vi "Experiment header-bundle parameters section wise.vi"(6 "Logging queue element":T1={"Imaging Protocol"=enum."Live Imaging", "Number of Trials"=0, "Frame Size"=100, "# Averaged frames"=0, "Dwell time (us)"=0.1, "Index of Z-plane"=0, "Timelapse?"=FALSE, "Logging process is active"=FALSE, "Speed logging enabled"=FALSE, "tdms file ref"=refnum, "path"=path "", "Trial Number"=0, "Expected # points acquired"=FALSE, "Manually stopped"=FALSE, "Last trial"=FALSE, "Ch0 data"=[], "Ch1 data"=[], "Image Time"=[], "Continuous Time"=[], "Points acquired"={"Ch0 last trial"=0, "Ch1 last trial"=0, "All trials"=0}, "HW Timings File"=refnum} {"Frame Size" items=["100X100"=100, "128X128"=128, "200X200"=200, "256X256"=256, "512X512"=512, "1024x1024"=1024, "2048x2048"=2048]; "Dwell time (us)" format="%#.6g"}, 7 "Update header\ninterface cluster ?":bool, 8 "error in (no error)":errorcluster, 9 "Experiment data folder path":path, 10 "AOL_Globals":T22={"Imaging Protocol"=enum."AOL Z-Stack", "Number of POI"=0, "Number of Miniscans"=0, "Number of Trials"=0, "Number of Cycles "=0, "# Averaged Frames"=0, "Laser power (%)"=0, "Pockels (V)"=0.0, "Acquisition Length (sec)"=0.0, "Fill time (us)"=0.0, "POI Dwell time (us)"=0.0, "Miniscan Dwell time per pixel (us)"=0.0, "PMT 1"=0.0, "PMT 2"=0.0, "Back Apperture (mA)"=200.0, "Frame Size"=0, "Center Frequency"=0.0, "Field of View (norm)"=0.0, "DwellTime (us)"=0.0, "Wavelength (nm)"=0.0, "Zoom"=0.0, "AOL Z"=0.0, "AOL Mode"=enum."Raster", "GridXY"=0.0, "GridZ"=0.0, "TriggerPeriod (sec)"=0.0, "Number of Pixels in Miniscan"=0, "Experiment folder path"=path "", "X centre"=0.0, "Y centre"=0.0, "Angle (degrees)"=0.0, "Plane Mode"=0, "Threshold"=[], "Regenerate Chirps"=FALSE, "Rectangle ROI length (pixels)"=0, "Rectangle ROI height (pixels)"=0, "AOD fill"=4900, "StartupDelay"=0, "Samples Wait after Trigger"=5080, "Slip Cycle"=600000, "Add Cycle"=TRUE, "Functional Mode"=enum."Point", "Z Start"=0.0, "Z Stop"=0.0, "# Planes"=0} {"Plane Mode" items=["XY Plane", "XZ Plane", "YZ Plane", "arbitraryplane"]; "Frame Size" items=["100X100"=100, "128X128"=128, "200X200"=200, "256X256"=256, "512X512"=512, "1024x1024"=1024, "2048x2048"=2048]; "Back Apperture (mA)" format="%#.6g"; "Pockels (V)" format="%#.6g"; "PMT 2" format="%#.6g"; "PMT 1" format="%#.6g"; "Angle (degrees)" format="%#.6g"; "POI Dwell time (us)" format="%#.6g"}, 11 "Header file sections":T5=enum."GLOBAL PARAMETERS") -> (0 "error out":errorcluster, 3 "All header parameters in":T6 {"VOLUME IMAGING"."Plane Mode" items=["XY Plane", "XZ Plane", "YZ Plane", "arbitraryplane"]; "VOLUME IMAGING"."Basic Image meta data"."Frame Size" items=["100X100"=100, "128X128"=128, "200X200"=200, "256X256"=256, "512X512"=512, "1024x1024"=1024, "2048x2048"=2048]; "AOL Z-STACK"."Hdr Basic Image meta data"."Frame Size" items=["100X100"=100, "128X128"=128, "200X200"=200, "256X256"=256, "512X512"=512, "1024x1024"=1024, "2048x2048"=2048]; "MOTOR Z-STACK"."Hdr Basic Image meta data"."Frame Size" items=["100X100"=100, "128X128"=128, "200X200"=200, "256X256"=256, "512X512"=512, "1024x1024"=1024, "2048x2048"=2048]; "FUNCTIONAL IMAGING"."Plane Mode" items=["XY Plane", "XZ Plane", "YZ Plane", "arbitraryplane"]; "FUNCTIONAL IMAGING"."Basic Image meta data"."Frame Size" items=["100X100"=100, "128X128"=128, "200X200"=200, "256X256"=256, "512X512"=512, "1024x1024"=1024, "2048x2048"=2048]; "TIME SERIES"."Basic Image meta data"."Frame Size" items=["100X100"=100, "128X128"=128, "200X200"=200, "256X256"=256, "512X512"=512, "1024x1024"=1024, "2048x2048"=2048]})   [LabVIEW 2017]
uses:
  Typedefs/Controls/AOL_Globals.ctl
  Typedefs/Imaging Protocols enum.ctl
  Typedefs/Frame Size.ctl
  Typedefs/AOL modes.ctl
  Typedefs/Plane Mode.ctl
  Typedefs/Functional Mode.ctl
  Typedefs/Header parameters cluster-ALL.ctl
  Typedefs/Header subclusters/Header params -Login.ctl
  Typedefs/Header subclusters/Header params-Global Parameters.ctl
  Misc/Experiment Type.ctl
  Typedefs/Header subclusters/Header params-Imaging Modes.ctl
  Typedefs/Header subclusters/Header params-Time Series.ctl
  Typedefs/Header subclusters/Header params-Basic image meta data.ctl
  Typedefs/Header subclusters/Header params-Motor Z-stack.ctl
  Typedefs/Header subclusters/Header params-AOL Z-stack.ctl
  Typedefs/Header subclusters/Header params-Functional Imaging.ctl
  Typedefs/Header subclusters/Header params-Calibration Setup.ctl
  Typedefs/Header subclusters/Header params-statistics.ctl
  Misc/Biology Information.ctl
  Typedefs/Header file sections.ctl
  Typedefs/Logging queue element.ctl
  Typedefs/Acquired points count.ctl
  Typedefs/Header subclusters/Header params-Volume Imaging.ctl
  Typedefs/Header file interface module functions enum.ctl
  Global Variables/General Globals.vi
  User profiles code/Globals/gl_UsrProfiles globals.vi
  Global Variables/gl_UI Ctrl Refs.vi
  Peripherals Control/Pockels/Globals/gl_Pockels control globals.vi
  Configuration code/Calibration/Globals/gl_Calibration globals.vi
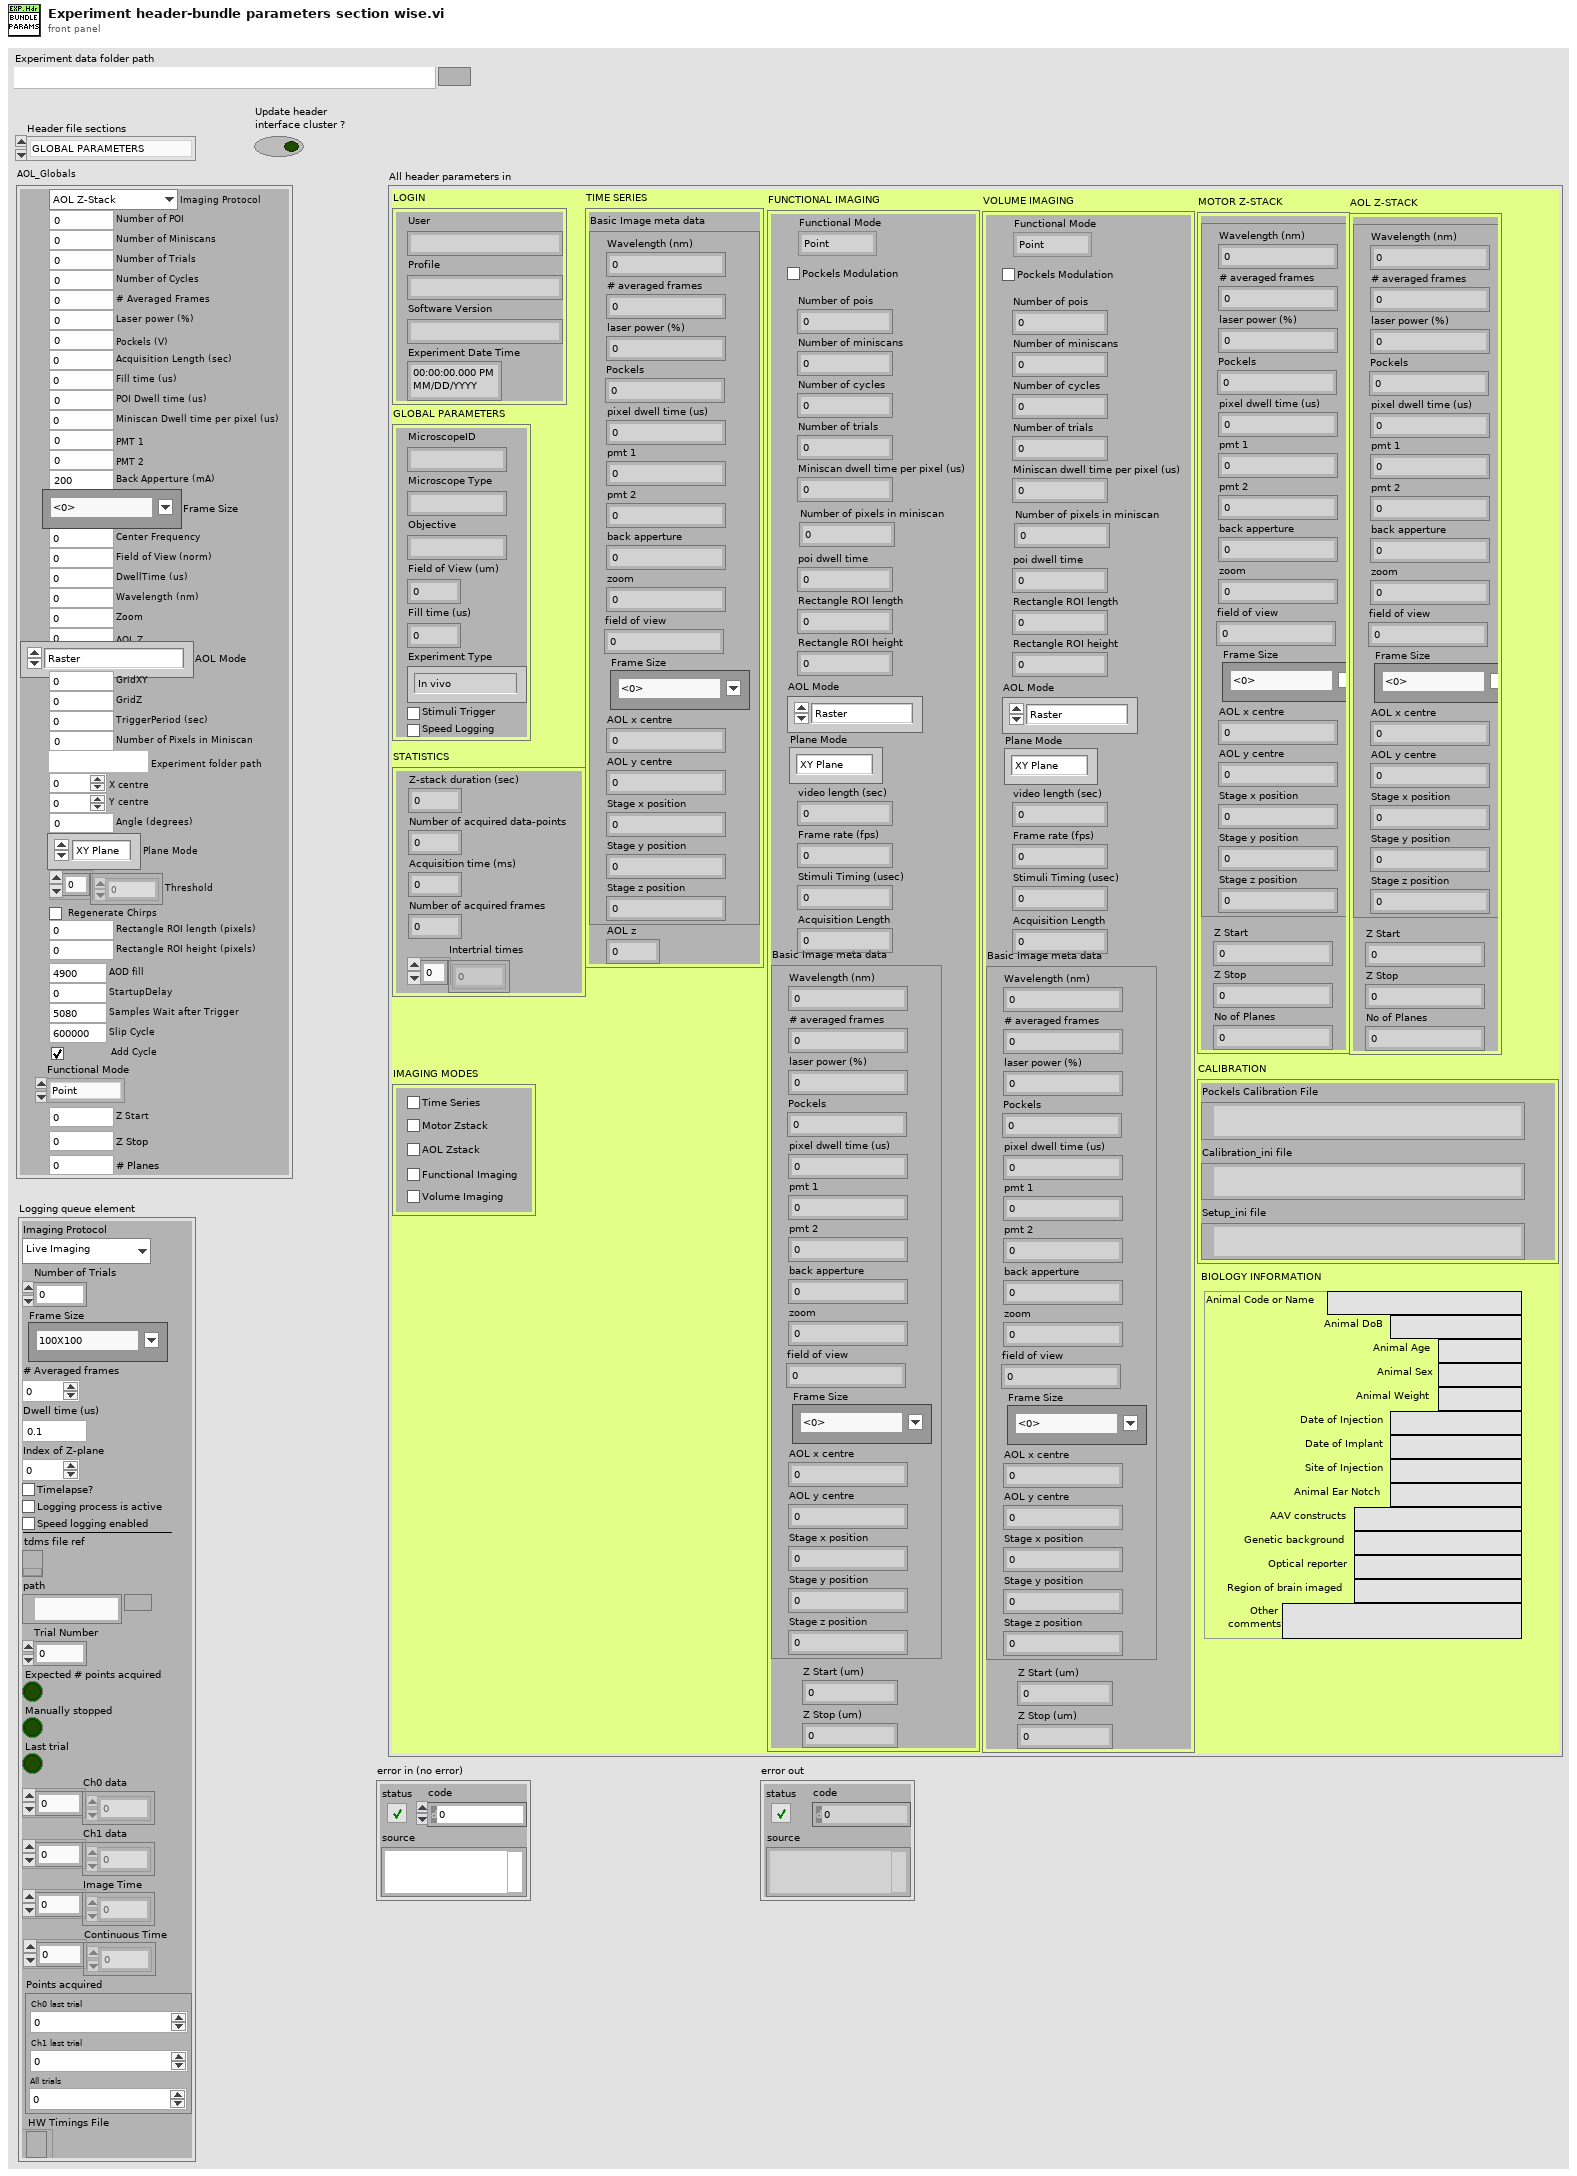
[diagram p1: front panel]
types:
  T1 = typedef "Logging queue element.ctl" = cluster{"Imaging Protocol":T2, "Number of Trials":u16, "Frame Size":T3, "# Averaged frames":u16, "Dwell time (us)":dbl, "Index of Z-plane":i32, "Timelapse?":bool, "Logging process is active":bool, "Speed logging enabled":bool, "tdms file ref":refnum<k34>, "path":path, "Trial Number":i32, "Expected # points acquired":bool, "Manually stopped":bool, "Last trial":bool, "Ch0 data":u32[], "Ch1 data":u32[], "Image Time":u64[], "Continuous Time":u64[], "Points acquired":T4, "HW Timings File":refnum<file>}
  T2 = typedef "Imaging Protocols enum.ctl" = enum16{"AOL Z-Stack", "Motor Z Stack", "Functional Acquisition", "Single Plane Acquisition", "Volume Acquisition", "Live Imaging", "Live Plane Imaging", "Live Volume Imaging"}
  T3 = typedef "Frame Size.ctl" = u16
  T4 = typedef "Acquired points count.ctl" = cluster{"Ch0 last trial":u64, "Ch1 last trial":u64, "All trials":u64}
  T5 = typedef "Header file sections.ctl" = enum16{"ALL SECTIONS", "LOGIN", "GLOBAL PARAMETERS", "IMAGING MODES", "TIME SERIES", "MOTOR Z-STACK", "AOL Z-STACK", "FUNCTIONAL IMAGING", "VOLUME IMAGING", "CALIBRATION", "STATISTICS", "BIOLOGY INFORMATION"}
  T6 = typedef "Header parameters cluster-ALL.ctl" = cluster{"LOGIN":T7, "GLOBAL PARAMETERS":T8, "IMAGING MODES":T10, "TIME SERIES":T11, "MOTOR Z-STACK ":T13, "AOL Z-STACK":T14, "FUNCTIONAL IMAGING":T15, "VOLUME IMAGING":T15, "CALIBRATION":T19, "STATISTICS":T20, "BIOLOGY INFORMATION":T21}
  T7 = typedef "Header params -Login.ctl" = cluster{"User":string, "Profile":string, "Software Version":string, "Experiment Date Time":timestamp}
  T8 = typedef "Header params-Global Parameters.ctl" = cluster{"MicroscopeID":string, "Microscope Type":string, "Objective":string, "Field of View (um)":dbl, "Fill time (us)":dbl, "Experiment Type":T9, "Stimuli Trigger":bool, "Speed Logging":bool}
  T9 = typedef "Experiment Type.ctl" = enum16{"In vivo", "In vitro", "Testing", "Calibration", "Other"}
  T10 = typedef "Header params-Imaging Modes.ctl" = cluster{"Time Series":bool, "Motor Zstack":bool, "AOL Zstack":bool, "Functional Imaging":bool, "Volume Imaging":bool}
  T11 = typedef "Header params-Time Series.ctl" = cluster{"Basic Image meta data":T12, "AOL z":dbl}
  T12 = typedef "Header params-Basic image meta data.ctl" = cluster{"Wavelength (nm)":dbl, "# averaged frames":dbl, "laser power (%)":dbl, "Pockels":dbl, "pixel dwell time (us)":dbl, "pmt 1":dbl, "pmt 2":dbl, "back apperture":dbl, "zoom":dbl, "field of view":dbl, "Frame Size":T3, "AOL x centre":dbl, "AOL y centre":dbl, "Stage x position":dbl, "Stage y position":dbl, "Stage z position":dbl}
  T13 = typedef "Header params-Motor Z-stack.ctl" = cluster{"Hdr Basic Image meta data":T12, "Z Start":dbl, "Z Stop":dbl, "No of Planes":i32}
  T14 = typedef "Header params-AOL Z-stack.ctl" = cluster{"Hdr Basic Image meta data":T12, "Z Start":dbl, "Z Stop":dbl, "No of Planes":i32}
  T15 = typedef "Header params-Functional Imaging.ctl" = cluster{"Functional Mode":T16, "Pockels Modulation":bool, "Number of pois":dbl, "Number of miniscans":dbl, "Number of cycles":dbl, "Number of trials":dbl, "Miniscan dwell time per pixel (us)":dbl, "Number of pixels in miniscan":dbl, "poi dwell time":dbl, "Rectangle ROI length":dbl, "Rectangle ROI height":dbl, "AOL Mode":T17, "Plane Mode":T18, "video length (sec)":dbl, "Frame rate (fps)":dbl, "Stimuli Timing (usec)":dbl, "Acquisition Length":dbl, "Basic Image meta data":T12, "Z Start (um)":dbl, "Z Stop (um)":dbl}
  T16 = typedef "Functional Mode.ctl" = enum16{"Point", "Line", "Patch", "Plane", "Volume"}
  T17 = typedef "AOL modes.ctl" = enum16{"Raster", "Structural", "Pointing", "Mini Scan", "Alignment"}
  T18 = typedef "Plane Mode.ctl" = u16
  T19 = typedef "Header params-Calibration Setup.ctl" = cluster{"Pockels Calibration File":path, "Calibration_ini file":path, "Setup_ini file":path}
  T20 = typedef "Header params-statistics.ctl" = cluster{"Z-stack duration (sec)":dbl, "Number of acquired data-points":dbl, "Acquisition time (ms)":dbl, "Number of acquired frames":dbl, "Intertrial times":dbl[]}
  T21 = typedef "Biology Information.ctl" = cluster{"Animal Code or Name":string, "Animal DoB":string, "Animal Age":string, "Animal Sex":string, "Animal Weight":string, "Date of Injection":string, "Date of Implant":string, "Site of Injection":string, "Animal Ear Notch":string, "AAV constructs":string, "Genetic background":string, "Optical reporter":string, "Region of brain imaged":string, "Other \ncomments":string}
  T22 = typedef "AOL_Globals.ctl" = cluster{"Imaging Protocol":T2, "Number of POI":u16, "Number of Miniscans":u16, "Number of Trials":u16, "Number of Cycles ":u64, "# Averaged Frames":u16, "Laser power (%)":u8, "Pockels (V)":dbl, "Acquisition Length (sec)":dbl, "Fill time (us)":dbl, "POI Dwell time (us)":dbl, "Miniscan Dwell time per pixel (us)":dbl, "PMT 1":dbl, "PMT 2":dbl, "Back Apperture (mA)":dbl, "Frame Size":T3, "Center Frequency":dbl, "Field of View (norm)":dbl, "DwellTime (us)":dbl, "Wavelength (nm)":dbl, "Zoom":dbl, "AOL Z":dbl, "AOL Mode":T17, "GridXY":dbl, "GridZ":dbl, "TriggerPeriod (sec)":dbl, "Number of Pixels in Miniscan":u16, "Experiment folder path":path, "X centre":dbl, "Y centre":dbl, "Angle (degrees)":dbl, "Plane Mode":T18, "Threshold":u16[], "Regenerate Chirps":bool, "Rectangle ROI length (pixels)":u16, "Rectangle ROI height (pixels)":u16, "AOD fill":u16, "StartupDelay":i32, "Samples Wait after Trigger":u16, "Slip Cycle":u32, "Add Cycle":bool, "Functional Mode":T16, "Z Start":dbl, "Z Stop":dbl, "# Planes":i32}
  T23 = typedef "Header params-Volume Imaging.ctl" = cluster{"Functional Mode":T16, "Pockels Modulation":bool, "Number of pois":dbl, "Number of miniscans":dbl, "Number of cycles":dbl, "Number of trials":dbl, "Miniscan dwell time per pixel (us)":dbl, "Number of pixels in miniscan":dbl, "poi dwell time":dbl, "Rectangle ROI length":dbl, "Rectangle ROI height":dbl, "AOL Mode":T17, "Plane Mode":T18, "video length (sec)":dbl, "Frame rate (fps)":dbl, "Stimuli Timing (usec)":dbl, "Acquisition Length":dbl, "Basic Image meta data":T12, "Z Start (um)":dbl, "Z Stop (um)":dbl}
  T24 = typedef "UI ctrl refs cluster.ctl" = cluster{"Top level VI path":path, "Top level VI ref":refnum<vi>, "User menu ref":refnum<k9>, "Sub Panel control":refnum<vi>, "Imaging Param Tab":refnum<vi>, "Occurrence-Start drivers":refnum<k4>, "Occurrence-Speed logging initialised":refnum<k4>, "Occurrence-XYZ stage initialised":refnum<k4>, "Exit button":refnum<vi>, "Status ind":refnum<vi>, "Set as origin":refnum<vi>, "Speed Logging":refnum<vi>, "Time Lapse":refnum<vi>, "Live Imaging":refnum<vi>, "AOL Z Stack":refnum<vi>, "Motor Z Stack":refnum<vi>, "Funct Acq button":refnum<vi>, "Hard Shutter":refnum<vi>, "Virtual Shutter":refnum<vi>, "Laser Power":refnum<vi>, "AOL Mode":refnum<vi>, "Frame Size":refnum<vi>, "Field of View":refnum<vi>, "Dwell Time":refnum<vi>, "Zoom":refnum<vi>, "AOL Z":refnum<vi>, "Objective":refnum<vi>, "Axis":refnum<vi>, "Paths & Names":refnum<vi>, "Experiment folder path (ind.)":refnum<vi>, "Last State (Ind.)":refnum<vi>, "Averages":refnum<vi>, "Angle (degrees)":refnum<vi>, "X centre":refnum<vi>, "Y centre":refnum<vi>, "Plane Mode":refnum<vi>, "# Planes":refnum<vi>, "Z Start":refnum<vi>, "Z Stop":refnum<vi>, "Z Step":refnum<vi>, "PMT 1":refnum<vi>, "PMT 2":refnum<vi>, "Stage XYZ Position":refnum<vi>, "Pockels@Z Start":refnum<vi>, "Pockels@Z Stop":refnum<vi>, "Obtain Z Start":refnum<vi>, "Obtain Z Stop":refnum<vi>, "Live stim.trig.period":refnum<vi>, "Live stim.trig.enable":refnum<vi>, "XY Stage Move":refnum<vi>, "Funct. Acq. Pockels Modulation":refnum<vi>, "Enable Video Recording":refnum<vi>, "Video Record-Live Imaging":refnum<vi>, "Video Record-Funct acq":refnum<vi>, "AOL Z-stack Chirps Ready (ind)":refnum<vi>, "Center freq ind (nm)":refnum<vi>, "Pickup mode (ind)":refnum<vi>, "Logging queue (ind)":refnum<vi>, "Back aperture power (ind.)":refnum<vi>, "Power after objective (ind.)":refnum<vi>, "Switch user":refnum<vi>, "Ls1 Conn. Status":refnum<vi>, "Ls1Tuning Status":refnum<vi>, "Ls1 Faults":refnum<vi>, "Ls1 Connection":refnum<vi>, "Ls1 Mode":refnum<vi>, "Ls1 POWER [mW]":refnum<vi>, "Ls1Shutter":refnum<vi>, "Ls1 Wavelength":refnum<vi>, "Ls1 Note":refnum<vi>, "Ls1 Confirm Wav":refnum<vi>, "Ls1 PreChrp Prism1":refnum<vi>, "Ls1 PreChrp Prism2":refnum<vi>, "Ls1 wav top Ind":refnum<vi>, "Ls1 power top Ind":refnum<vi>, "Ls1 Pump peak Hold":refnum<vi>, "Ls1 Status Ind":refnum<vi>, "Ls1 wav cancel":refnum<vi>, "Experiment Type":refnum<vi>, "Biology Information":refnum<vi>}
  T25 = typedef "Header file interface module functions enum.ctl" = enum16{"Load experiment header file", "Save experiment header file", "Clear stored values", "Read stored values", "Update specific value in memory", "Update values in memory"}
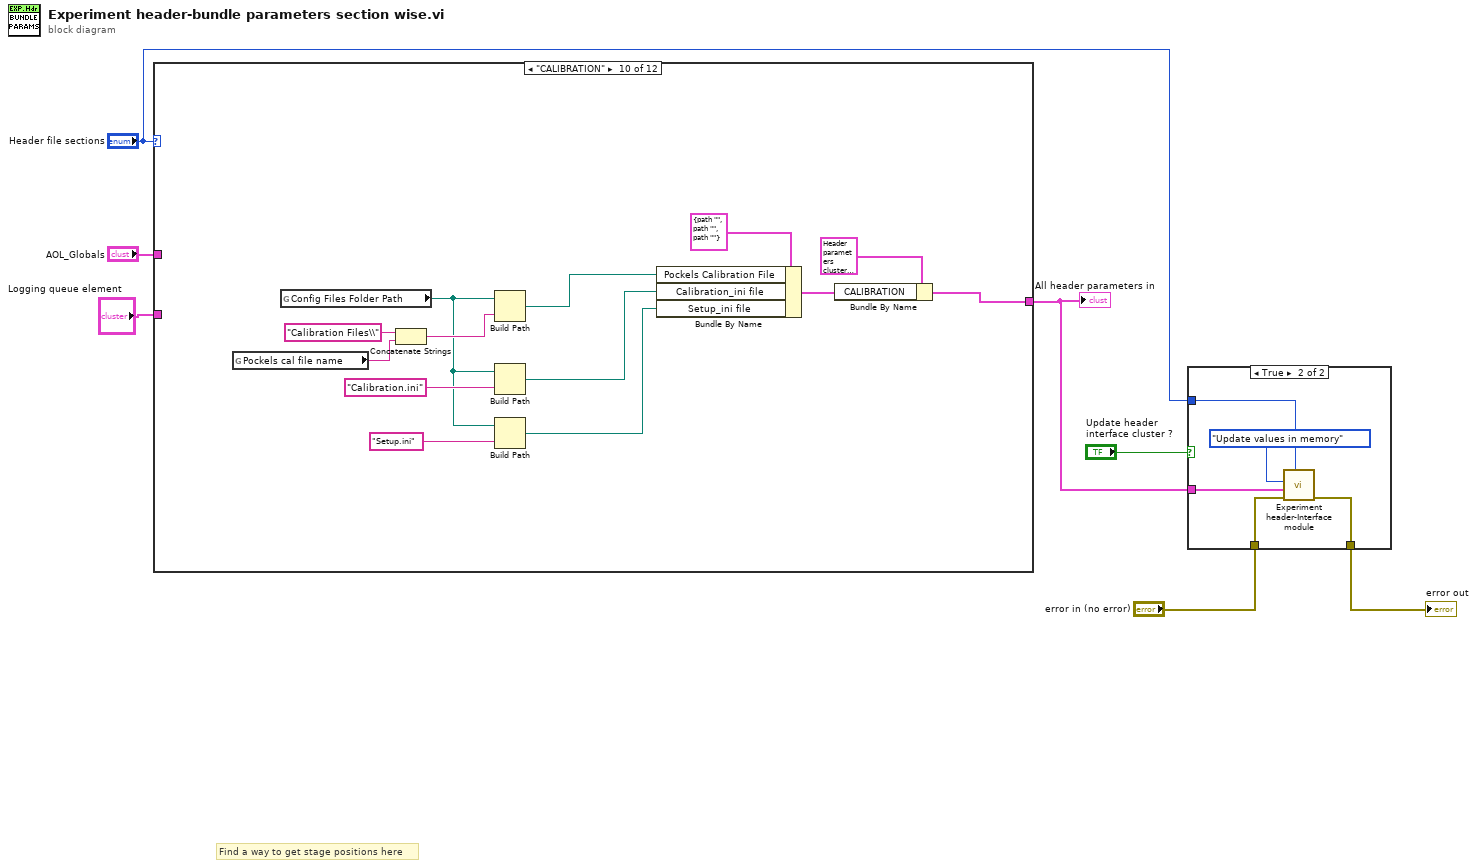
[diagram p0: block diagram]
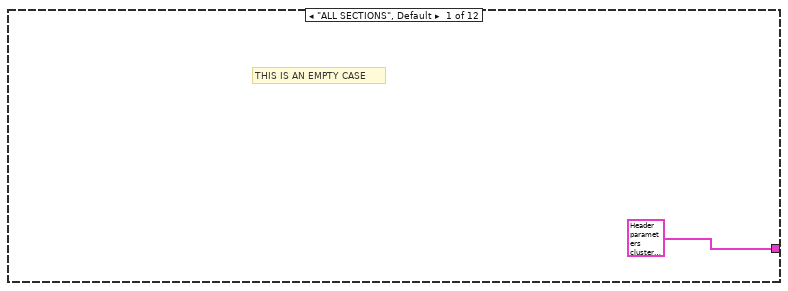
[diagram p3: hidden frame]
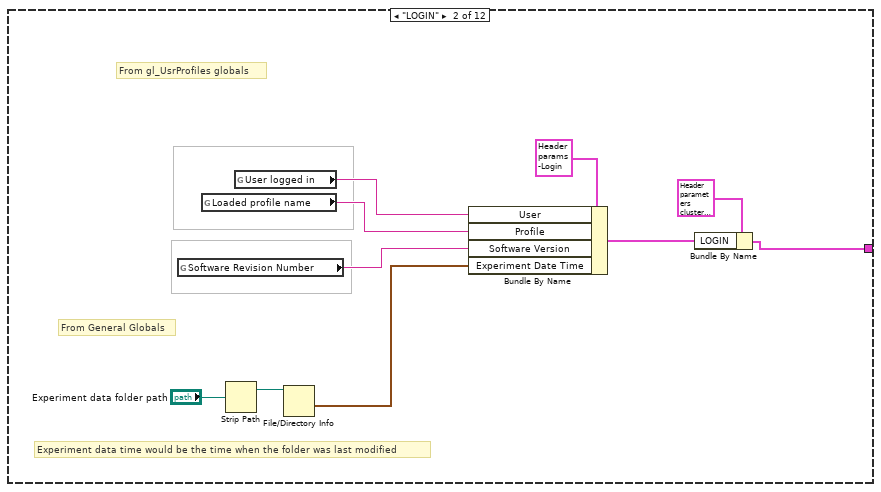
[diagram p4: hidden frame]
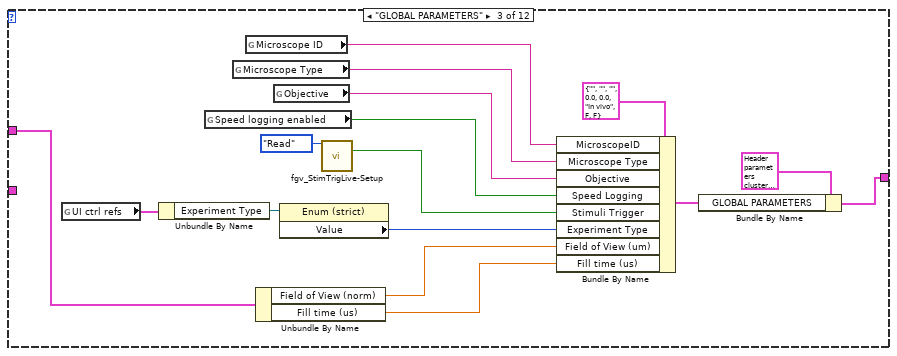
[diagram p5: hidden frame]
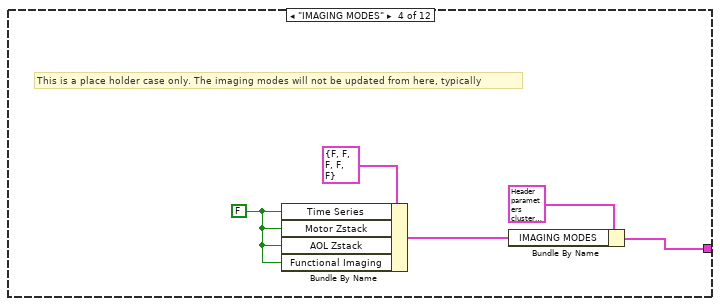
[diagram p6: hidden frame]
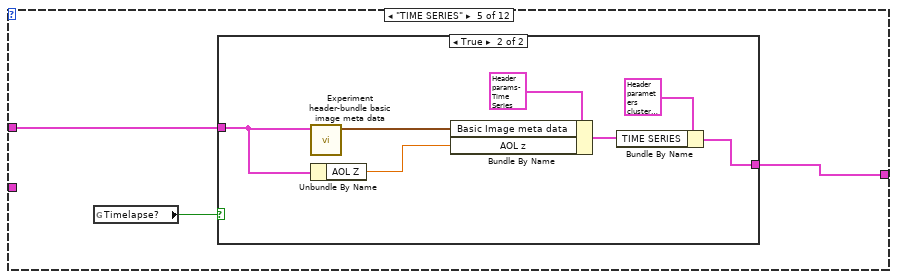
[diagram p7: hidden frame]
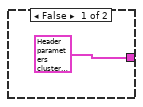
[diagram p8: hidden frame]
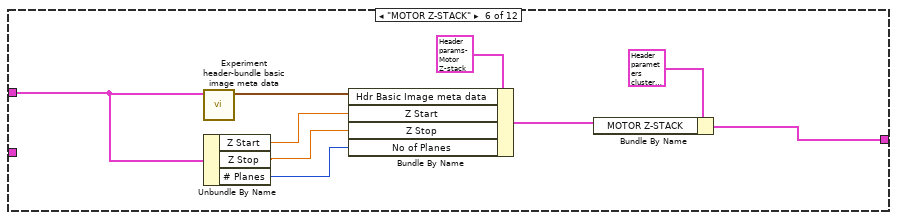
[diagram p9: hidden frame]
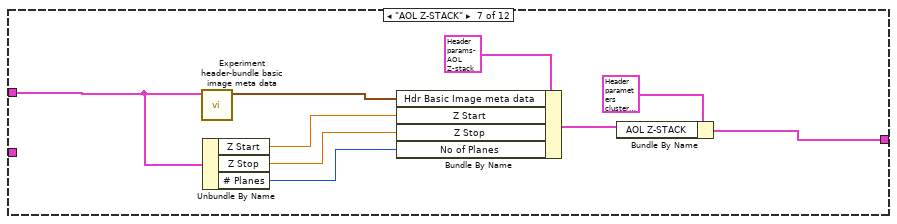
[diagram p10: hidden frame]
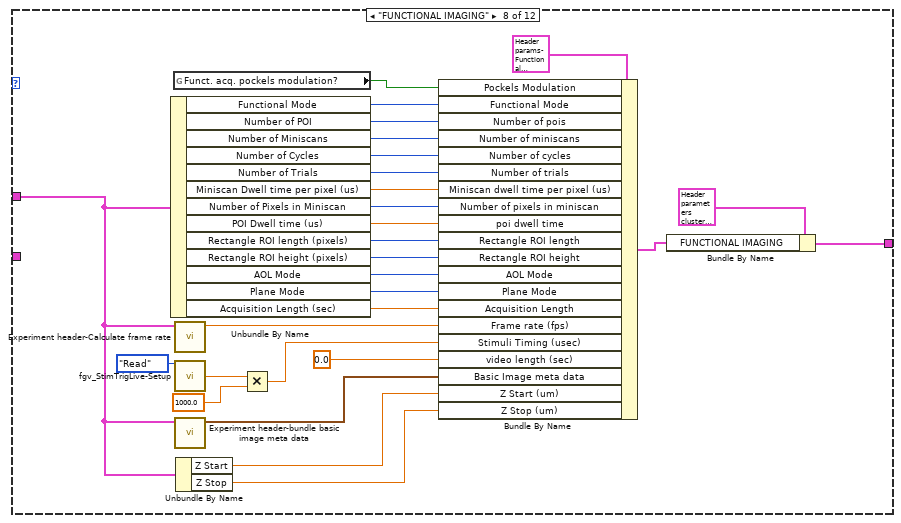
[diagram p11: hidden frame]
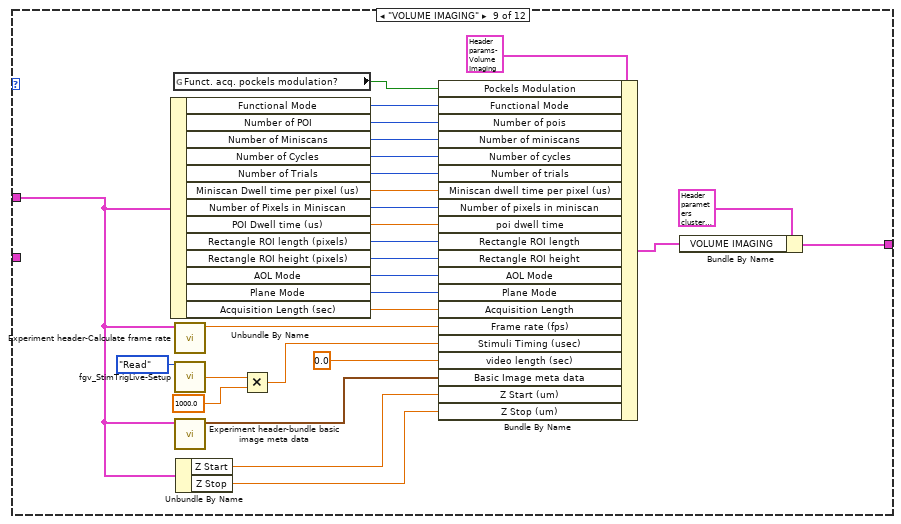
[diagram p12: hidden frame]
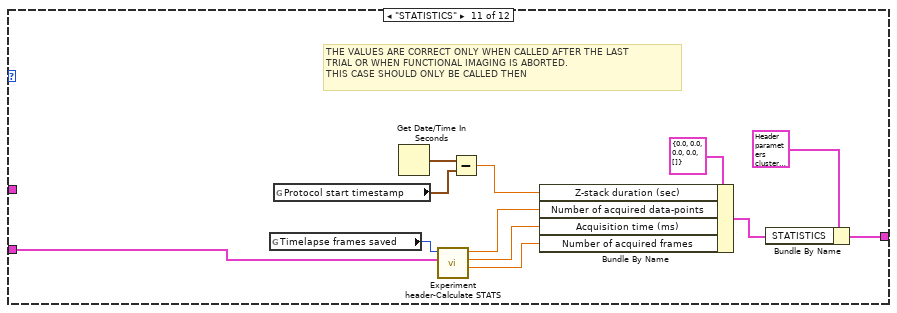
[diagram p13: hidden frame]
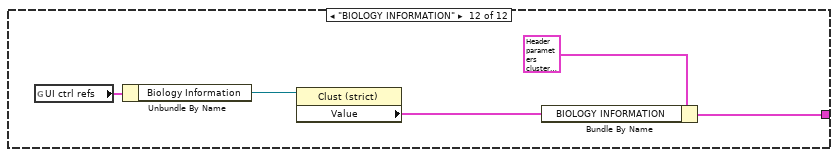
[diagram p14: hidden frame]
diagram:
  # "Find a way to get stage positions here"
  n1 = case shown="\"CALIBRATION\"" "Header file sections" {
    tunnel: "AOL_Globals" -> [_ _ w30 _ w41 w54 w63 w71 w100 _ _ _]
    tunnel: [T6 {"LOGIN"={"User"="Olympus  20X", "Profile"="", "Software Version"="", "Experiment Date Time"=timestamp(0 s since 1904-01-01)}, "GLOBAL PARAMETERS"={"MicroscopeID"="", "Microscope Type"="", "Objective"="", "Field of View (um)"=0.0, "Fill time (us)"=0.0, "Experiment Type"=enum."In vivo", "Stimuli Trigger"=FALSE, "Speed Logging"=FALSE}, "IMAGING MODES"={"Time Series"=FALSE, "Motor Zstack"=FALSE, "AOL Zstack"=FALSE, "Functional Imaging"=FALSE, "Volume Imaging"=FALSE}, "TIME SERIES"={"Basic Image meta data"={"Wavelength (nm)"=0.0, "# averaged frames"=0.0, "laser power (%)"=0.0, "Pockels"=0.0, "pixel dwell time (us)"=0.0, "pmt 1"=0.0, "pmt 2"=0.0, "back apperture"=0.0, "zoom"=0.0, "field of view"=0.0, "Frame Size"=0, "AOL x centre"=0.0, "AOL y centre"=0.0, "Stage x position"=0.0, "Stage y position"=0.0, "Stage z position"=0.0}, "AOL z"=0.0}, "MOTOR Z-STACK "={"Hdr Basic Image meta data"={"Wavelength (nm)"=0.0, "# averaged frames"=0.0, "laser power (%)"=0.0, "Pockels"=0.0, "pixel dwell time (us)"=0.0, "pmt 1"=0.0, "pmt 2"=0.0, "back apperture"=0.0, "zoom"=0.0, "field of view"=0.0, "Frame Size"=0, "AOL x centre"=0.0, "AOL y centre"=0.0, "Stage x position"=0.0, "Stage y position"=0.0, "Stage z position"=0.0}, "Z Start"=0.0, "Z Stop"=0.0, "No of Planes"=0}, "AOL Z-STACK"={"Hdr Basic Image meta data"={"Wavelength (nm)"=0.0, "# averaged frames"=0.0, "laser power (%)"=0.0, "Pockels"=0.0, "pixel dwell time (us)"=0.0, "pmt 1"=0.0, "pmt 2"=0.0, "back apperture"=0.0, "zoom"=0.0, "field of view"=0.0, "Frame Size"=0, "AOL x centre"=0.0, "AOL y centre"=0.0, "Stage x position"=0.0, "Stage y position"=0.0, "Stage z position"=0.0}, "Z Start"=0.0, "Z Stop"=0.0, "No of Planes"=0}, "FUNCTIONAL IMAGING"={"Functional Mode"=enum."Point", "Pockels Modulation"=FALSE, "Number of pois"=0.0, "Number of miniscans"=0.0, "Number of cycles"=0.0, "Number of trials"=0.0, "Miniscan dwell time per pixel (us)"=0.0, "Number of pixels in miniscan"=0.0, "poi dwell time"=0.0, "Rectangle ROI length"=0.0, "Rectangle ROI height"=0.0, "AOL Mode"=enum."Raster", "Plane Mode"=0, "video length (sec)"=0.0, "Frame rate (fps)"=0.0, "Stimuli Timing (usec)"=0.0, "Acquisition Length"=0.0, "Basic Image meta data"={"Wavelength (nm)"=0.0, "# averaged frames"=0.0, "laser power (%)"=0.0, "Pockels"=0.0, "pixel dwell time (us)"=0.0, "pmt 1"=0.0, "pmt 2"=0.0, "back apperture"=0.0, "zoom"=0.0, "field of view"=0.0, "Frame Size"=0, "AOL x centre"=0.0, "AOL y centre"=0.0, "Stage x position"=0.0, "Stage y position"=0.0, "Stage z position"=0.0}, "Z Start (um)"=0.0, "Z Stop (um)"=0.0}, "VOLUME IMAGING"={"Functional Mode"=enum."Point", "Pockels Modulation"=FALSE, "Number of pois"=0.0, "Number of miniscans"=0.0, "Number of cycles"=0.0, "Number of trials"=0.0, "Miniscan dwell time per pixel (us)"=0.0, "Number of pixels in miniscan"=0.0, "poi dwell time"=0.0, "Rectangle ROI length"=0.0, "Rectangle ROI height"=0.0, "AOL Mode"=enum."Raster", "Plane Mode"=0, "video length (sec)"=0.0, "Frame rate (fps)"=0.0, "Stimuli Timing (usec)"=0.0, "Acquisition Length"=0.0, "Basic Image meta data"={"Wavelength (nm)"=0.0, "# averaged frames"=0.0, "laser power (%)"=0.0, "Pockels"=0.0, "pixel dwell time (us)"=0.0, "pmt 1"=0.0, "pmt 2"=0.0, "back apperture"=0.0, "zoom"=0.0, "field of view"=0.0, "Frame Size"=0, "AOL x centre"=0.0, "AOL y centre"=0.0, "Stage x position"=0.0, "Stage y position"=0.0, "Stage z position"=0.0}, "Z Start (um)"=0.0, "Z Stop (um)"=0.0}, "CALIBRATION"={"Pockels Calibration File"=path "", "Calibration_ini file"=path "", "Setup_ini file"=path ""}, "STATISTICS"={"Z-stack duration (sec)"=0.0, "Number of acquired data-points"=0.0, "Acquisition time (ms)"=0.0, "Number of acquired frames"=0.0, "Intertrial times"=[]}, "BIOLOGY INFORMATION"={"Animal Code or Name"="", "Animal DoB"="", "Animal Age"="", "Animal Sex"="", "Animal Weight"="", "Date of Injection"="", "Date of Implant"="", "Site of Injection"="", "Animal Ear Notch"="", "AAV constructs"="", "Genetic background"="", "Optical reporter"="", "Region of brain imaged"="", "Other \ncomments"=""}} ("All header parameters in") w12 w19 w35 w42 w55 w66 w93 w122 w125 w148 w150] -> w6
    tunnel: "Logging queue element" -> [_ _ _ _ _ _ _ _ _ _ w146 _]
    frame "ALL SECTIONS", Default {
      # "THIS IS AN EMPTY CASE"
    }
    frame "LOGIN" {
      # "Experiment data time would be the time when the folder was last modified"
      # "From General Globals"
      # "From gl_UsrProfiles globals"
      n2 = global read "General Globals.vi" "Software Revision Number"() -> (w15:string)
      n3 = global read "gl_UsrProfiles globals.vi" "Loaded profile name"() -> (w16:string)
      n4 = Strip Path(path="Experiment data folder path") -> (stripped path=w10:path)  [unwired: 1 out]
      n5 = global read "gl_UsrProfiles globals.vi" "User logged in"() -> (w17:string)
      n6 = File/Directory Info(path=w10) -> (last mod=w9:timestamp)  [unwired: 1 in, 6 out]
      n7 = Bundle By Name(cluster=T7 {"User"="", "Profile"="", "Software Version"="", "Experiment Date Time"=timestamp(0 s since 1904-01-01)} ("LOGIN"), "User"=w17, "Profile"=w16, "Software Version"=w15, "Experiment Date Time"=w9) -> (w13:T7)
      n8 = Bundle By Name(cluster=T6 {"LOGIN"={"User"="Olympus  20X", "Profile"="", "Software Version"="", "Experiment Date Time"=timestamp(0 s since 1904-01-01)}, "GLOBAL PARAMETERS"={"MicroscopeID"="", "Microscope Type"="", "Objective"="", "Field of View (um)"=0.0, "Fill time (us)"=0.0, "Experiment Type"=enum."In vivo", "Stimuli Trigger"=FALSE, "Speed Logging"=FALSE}, "IMAGING MODES"={"Time Series"=FALSE, "Motor Zstack"=FALSE, "AOL Zstack"=FALSE, "Functional Imaging"=FALSE, "Volume Imaging"=FALSE}, "TIME SERIES"={"Basic Image meta data"={"Wavelength (nm)"=0.0, "# averaged frames"=0.0, "laser power (%)"=0.0, "Pockels"=0.0, "pixel dwell time (us)"=0.0, "pmt 1"=0.0, "pmt 2"=0.0, "back apperture"=0.0, "zoom"=0.0, "field of view"=0.0, "Frame Size"=0, "AOL x centre"=0.0, "AOL y centre"=0.0, "Stage x position"=0.0, "Stage y position"=0.0, "Stage z position"=0.0}, "AOL z"=0.0}, "MOTOR Z-STACK "={"Hdr Basic Image meta data"={"Wavelength (nm)"=0.0, "# averaged frames"=0.0, "laser power (%)"=0.0, "Pockels"=0.0, "pixel dwell time (us)"=0.0, "pmt 1"=0.0, "pmt 2"=0.0, "back apperture"=0.0, "zoom"=0.0, "field of view"=0.0, "Frame Size"=0, "AOL x centre"=0.0, "AOL y centre"=0.0, "Stage x position"=0.0, "Stage y position"=0.0, "Stage z position"=0.0}, "Z Start"=0.0, "Z Stop"=0.0, "No of Planes"=0}, "AOL Z-STACK"={"Hdr Basic Image meta data"={"Wavelength (nm)"=0.0, "# averaged frames"=0.0, "laser power (%)"=0.0, "Pockels"=0.0, "pixel dwell time (us)"=0.0, "pmt 1"=0.0, "pmt 2"=0.0, "back apperture"=0.0, "zoom"=0.0, "field of view"=0.0, "Frame Size"=0, "AOL x centre"=0.0, "AOL y centre"=0.0, "Stage x position"=0.0, "Stage y position"=0.0, "Stage z position"=0.0}, "Z Start"=0.0, "Z Stop"=0.0, "No of Planes"=0}, "FUNCTIONAL IMAGING"={"Functional Mode"=enum."Point", "Pockels Modulation"=FALSE, "Number of pois"=0.0, "Number of miniscans"=0.0, "Number of cycles"=0.0, "Number of trials"=0.0, "Miniscan dwell time per pixel (us)"=0.0, "Number of pixels in miniscan"=0.0, "poi dwell time"=0.0, "Rectangle ROI length"=0.0, "Rectangle ROI height"=0.0, "AOL Mode"=enum."Raster", "Plane Mode"=0, "video length (sec)"=0.0, "Frame rate (fps)"=0.0, "Stimuli Timing (usec)"=0.0, "Acquisition Length"=0.0, "Basic Image meta data"={"Wavelength (nm)"=0.0, "# averaged frames"=0.0, "laser power (%)"=0.0, "Pockels"=0.0, "pixel dwell time (us)"=0.0, "pmt 1"=0.0, "pmt 2"=0.0, "back apperture"=0.0, "zoom"=0.0, "field of view"=0.0, "Frame Size"=0, "AOL x centre"=0.0, "AOL y centre"=0.0, "Stage x position"=0.0, "Stage y position"=0.0, "Stage z position"=0.0}, "Z Start (um)"=0.0, "Z Stop (um)"=0.0}, "VOLUME IMAGING"={"Functional Mode"=enum."Point", "Pockels Modulation"=FALSE, "Number of pois"=0.0, "Number of miniscans"=0.0, "Number of cycles"=0.0, "Number of trials"=0.0, "Miniscan dwell time per pixel (us)"=0.0, "Number of pixels in miniscan"=0.0, "poi dwell time"=0.0, "Rectangle ROI length"=0.0, "Rectangle ROI height"=0.0, "AOL Mode"=enum."Raster", "Plane Mode"=0, "video length (sec)"=0.0, "Frame rate (fps)"=0.0, "Stimuli Timing (usec)"=0.0, "Acquisition Length"=0.0, "Basic Image meta data"={"Wavelength (nm)"=0.0, "# averaged frames"=0.0, "laser power (%)"=0.0, "Pockels"=0.0, "pixel dwell time (us)"=0.0, "pmt 1"=0.0, "pmt 2"=0.0, "back apperture"=0.0, "zoom"=0.0, "field of view"=0.0, "Frame Size"=0, "AOL x centre"=0.0, "AOL y centre"=0.0, "Stage x position"=0.0, "Stage y position"=0.0, "Stage z position"=0.0}, "Z Start (um)"=0.0, "Z Stop (um)"=0.0}, "CALIBRATION"={"Pockels Calibration File"=path "", "Calibration_ini file"=path "", "Setup_ini file"=path ""}, "STATISTICS"={"Z-stack duration (sec)"=0.0, "Number of acquired data-points"=0.0, "Acquisition time (ms)"=0.0, "Number of acquired frames"=0.0, "Intertrial times"=[]}, "BIOLOGY INFORMATION"={"Animal Code or Name"="", "Animal DoB"="", "Animal Age"="", "Animal Sex"="", "Animal Weight"="", "Date of Injection"="", "Date of Implant"="", "Site of Injection"="", "Animal Ear Notch"="", "AAV constructs"="", "Genetic background"="", "Optical reporter"="", "Region of brain imaged"="", "Other \ncomments"=""}} ("All header parameters in"), "LOGIN"=w13) -> (w12:T6)
    }
    frame "GLOBAL PARAMETERS" {
      n9 = global read "gl_UI Ctrl Refs.vi" "UI ctrl refs"() -> (w26:T24)
      n10 = Unbundle By Name(w26) -> ("Experiment Type"=w25:refnum<vi>)
      n11 = global read "General Globals.vi" "Speed logging enabled"() -> (w29:bool)
      n12 = global read "General Globals.vi" "Microscope Type"() -> (w32:string)
      n13 = global read "General Globals.vi" "Microscope ID"() -> (w33:string)
      n14 = Unbundle By Name(w30) -> ("Field of View (norm)"=w23:dbl, "Fill time (us)"=w22:dbl)
      n15 = global read "General Globals.vi" "Objective"() -> (w31:string)
      n16 = property class="Enum (strict)"(reference=w25) -> ("Value"=w24:T9)  [unwired: 1 in, 2 out]
      n17 = call "fgv_StimTrigLive-Setup.vi"("Function"=enum16{"Intialize", "Write", "Read", "Clear"}."Read") -> ("Live stim.trig.enable"=w27:bool)  [unwired: 11 in, 3 out]
      n18 = Bundle By Name(cluster=T8 {"MicroscopeID"="", "Microscope Type"="", "Objective"="", "Field of View (um)"=0.0, "Fill time (us)"=0.0, "Experiment Type"=enum."In vivo", "Stimuli Trigger"=FALSE, "Speed Logging"=FALSE} ("GLOBAL PARAMETERS"), "MicroscopeID"=w33, "Microscope Type"=w32, "Objective"=w31, "Speed Logging"=w29, "Stimuli Trigger"=w27, "Experiment Type"=w24, "Field of View (um)"=w23, "Fill time (us)"=w22) -> (w20:T8)
      n19 = Bundle By Name(cluster=T6 {"LOGIN"={"User"="Olympus  20X", "Profile"="", "Software Version"="", "Experiment Date Time"=timestamp(0 s since 1904-01-01)}, "GLOBAL PARAMETERS"={"MicroscopeID"="", "Microscope Type"="", "Objective"="", "Field of View (um)"=0.0, "Fill time (us)"=0.0, "Experiment Type"=enum."In vivo", "Stimuli Trigger"=FALSE, "Speed Logging"=FALSE}, "IMAGING MODES"={"Time Series"=FALSE, "Motor Zstack"=FALSE, "AOL Zstack"=FALSE, "Functional Imaging"=FALSE, "Volume Imaging"=FALSE}, "TIME SERIES"={"Basic Image meta data"={"Wavelength (nm)"=0.0, "# averaged frames"=0.0, "laser power (%)"=0.0, "Pockels"=0.0, "pixel dwell time (us)"=0.0, "pmt 1"=0.0, "pmt 2"=0.0, "back apperture"=0.0, "zoom"=0.0, "field of view"=0.0, "Frame Size"=0, "AOL x centre"=0.0, "AOL y centre"=0.0, "Stage x position"=0.0, "Stage y position"=0.0, "Stage z position"=0.0}, "AOL z"=0.0}, "MOTOR Z-STACK "={"Hdr Basic Image meta data"={"Wavelength (nm)"=0.0, "# averaged frames"=0.0, "laser power (%)"=0.0, "Pockels"=0.0, "pixel dwell time (us)"=0.0, "pmt 1"=0.0, "pmt 2"=0.0, "back apperture"=0.0, "zoom"=0.0, "field of view"=0.0, "Frame Size"=0, "AOL x centre"=0.0, "AOL y centre"=0.0, "Stage x position"=0.0, "Stage y position"=0.0, "Stage z position"=0.0}, "Z Start"=0.0, "Z Stop"=0.0, "No of Planes"=0}, "AOL Z-STACK"={"Hdr Basic Image meta data"={"Wavelength (nm)"=0.0, "# averaged frames"=0.0, "laser power (%)"=0.0, "Pockels"=0.0, "pixel dwell time (us)"=0.0, "pmt 1"=0.0, "pmt 2"=0.0, "back apperture"=0.0, "zoom"=0.0, "field of view"=0.0, "Frame Size"=0, "AOL x centre"=0.0, "AOL y centre"=0.0, "Stage x position"=0.0, "Stage y position"=0.0, "Stage z position"=0.0}, "Z Start"=0.0, "Z Stop"=0.0, "No of Planes"=0}, "FUNCTIONAL IMAGING"={"Functional Mode"=enum."Point", "Pockels Modulation"=FALSE, "Number of pois"=0.0, "Number of miniscans"=0.0, "Number of cycles"=0.0, "Number of trials"=0.0, "Miniscan dwell time per pixel (us)"=0.0, "Number of pixels in miniscan"=0.0, "poi dwell time"=0.0, "Rectangle ROI length"=0.0, "Rectangle ROI height"=0.0, "AOL Mode"=enum."Raster", "Plane Mode"=0, "video length (sec)"=0.0, "Frame rate (fps)"=0.0, "Stimuli Timing (usec)"=0.0, "Acquisition Length"=0.0, "Basic Image meta data"={"Wavelength (nm)"=0.0, "# averaged frames"=0.0, "laser power (%)"=0.0, "Pockels"=0.0, "pixel dwell time (us)"=0.0, "pmt 1"=0.0, "pmt 2"=0.0, "back apperture"=0.0, "zoom"=0.0, "field of view"=0.0, "Frame Size"=0, "AOL x centre"=0.0, "AOL y centre"=0.0, "Stage x position"=0.0, "Stage y position"=0.0, "Stage z position"=0.0}, "Z Start (um)"=0.0, "Z Stop (um)"=0.0}, "VOLUME IMAGING"={"Functional Mode"=enum."Point", "Pockels Modulation"=FALSE, "Number of pois"=0.0, "Number of miniscans"=0.0, "Number of cycles"=0.0, "Number of trials"=0.0, "Miniscan dwell time per pixel (us)"=0.0, "Number of pixels in miniscan"=0.0, "poi dwell time"=0.0, "Rectangle ROI length"=0.0, "Rectangle ROI height"=0.0, "AOL Mode"=enum."Raster", "Plane Mode"=0, "video length (sec)"=0.0, "Frame rate (fps)"=0.0, "Stimuli Timing (usec)"=0.0, "Acquisition Length"=0.0, "Basic Image meta data"={"Wavelength (nm)"=0.0, "# averaged frames"=0.0, "laser power (%)"=0.0, "Pockels"=0.0, "pixel dwell time (us)"=0.0, "pmt 1"=0.0, "pmt 2"=0.0, "back apperture"=0.0, "zoom"=0.0, "field of view"=0.0, "Frame Size"=0, "AOL x centre"=0.0, "AOL y centre"=0.0, "Stage x position"=0.0, "Stage y position"=0.0, "Stage z position"=0.0}, "Z Start (um)"=0.0, "Z Stop (um)"=0.0}, "CALIBRATION"={"Pockels Calibration File"=path "", "Calibration_ini file"=path "", "Setup_ini file"=path ""}, "STATISTICS"={"Z-stack duration (sec)"=0.0, "Number of acquired data-points"=0.0, "Acquisition time (ms)"=0.0, "Number of acquired frames"=0.0, "Intertrial times"=[]}, "BIOLOGY INFORMATION"={"Animal Code or Name"="", "Animal DoB"="", "Animal Age"="", "Animal Sex"="", "Animal Weight"="", "Date of Injection"="", "Date of Implant"="", "Site of Injection"="", "Animal Ear Notch"="", "AAV constructs"="", "Genetic background"="", "Optical reporter"="", "Region of brain imaged"="", "Other \ncomments"=""}} ("All header parameters in"), "GLOBAL PARAMETERS"=w20) -> (w19:T6)
    }
    frame "IMAGING MODES" {
      w38 = FALSE ("Time Series")
      # "This is a place holder case only. The imaging modes will not be updated from here, typically"
      n20 = Bundle By Name(cluster=T10 {"Time Series"=FALSE, "Motor Zstack"=FALSE, "AOL Zstack"=FALSE, "Functional Imaging"=FALSE, "Volume Imaging"=FALSE} ("IMAGING MODES"), "Time Series"=w38, "Motor Zstack"=w38, "AOL Zstack"=w38, "Functional Imaging"=w38) -> (w36:T10)
      n21 = Bundle By Name(cluster=T6 {"LOGIN"={"User"="Olympus  20X", "Profile"="", "Software Version"="", "Experiment Date Time"=timestamp(0 s since 1904-01-01)}, "GLOBAL PARAMETERS"={"MicroscopeID"="", "Microscope Type"="", "Objective"="", "Field of View (um)"=0.0, "Fill time (us)"=0.0, "Experiment Type"=enum."In vivo", "Stimuli Trigger"=FALSE, "Speed Logging"=FALSE}, "IMAGING MODES"={"Time Series"=FALSE, "Motor Zstack"=FALSE, "AOL Zstack"=FALSE, "Functional Imaging"=FALSE, "Volume Imaging"=FALSE}, "TIME SERIES"={"Basic Image meta data"={"Wavelength (nm)"=0.0, "# averaged frames"=0.0, "laser power (%)"=0.0, "Pockels"=0.0, "pixel dwell time (us)"=0.0, "pmt 1"=0.0, "pmt 2"=0.0, "back apperture"=0.0, "zoom"=0.0, "field of view"=0.0, "Frame Size"=0, "AOL x centre"=0.0, "AOL y centre"=0.0, "Stage x position"=0.0, "Stage y position"=0.0, "Stage z position"=0.0}, "AOL z"=0.0}, "MOTOR Z-STACK "={"Hdr Basic Image meta data"={"Wavelength (nm)"=0.0, "# averaged frames"=0.0, "laser power (%)"=0.0, "Pockels"=0.0, "pixel dwell time (us)"=0.0, "pmt 1"=0.0, "pmt 2"=0.0, "back apperture"=0.0, "zoom"=0.0, "field of view"=0.0, "Frame Size"=0, "AOL x centre"=0.0, "AOL y centre"=0.0, "Stage x position"=0.0, "Stage y position"=0.0, "Stage z position"=0.0}, "Z Start"=0.0, "Z Stop"=0.0, "No of Planes"=0}, "AOL Z-STACK"={"Hdr Basic Image meta data"={"Wavelength (nm)"=0.0, "# averaged frames"=0.0, "laser power (%)"=0.0, "Pockels"=0.0, "pixel dwell time (us)"=0.0, "pmt 1"=0.0, "pmt 2"=0.0, "back apperture"=0.0, "zoom"=0.0, "field of view"=0.0, "Frame Size"=0, "AOL x centre"=0.0, "AOL y centre"=0.0, "Stage x position"=0.0, "Stage y position"=0.0, "Stage z position"=0.0}, "Z Start"=0.0, "Z Stop"=0.0, "No of Planes"=0}, "FUNCTIONAL IMAGING"={"Functional Mode"=enum."Point", "Pockels Modulation"=FALSE, "Number of pois"=0.0, "Number of miniscans"=0.0, "Number of cycles"=0.0, "Number of trials"=0.0, "Miniscan dwell time per pixel (us)"=0.0, "Number of pixels in miniscan"=0.0, "poi dwell time"=0.0, "Rectangle ROI length"=0.0, "Rectangle ROI height"=0.0, "AOL Mode"=enum."Raster", "Plane Mode"=0, "video length (sec)"=0.0, "Frame rate (fps)"=0.0, "Stimuli Timing (usec)"=0.0, "Acquisition Length"=0.0, "Basic Image meta data"={"Wavelength (nm)"=0.0, "# averaged frames"=0.0, "laser power (%)"=0.0, "Pockels"=0.0, "pixel dwell time (us)"=0.0, "pmt 1"=0.0, "pmt 2"=0.0, "back apperture"=0.0, "zoom"=0.0, "field of view"=0.0, "Frame Size"=0, "AOL x centre"=0.0, "AOL y centre"=0.0, "Stage x position"=0.0, "Stage y position"=0.0, "Stage z position"=0.0}, "Z Start (um)"=0.0, "Z Stop (um)"=0.0}, "VOLUME IMAGING"={"Functional Mode"=enum."Point", "Pockels Modulation"=FALSE, "Number of pois"=0.0, "Number of miniscans"=0.0, "Number of cycles"=0.0, "Number of trials"=0.0, "Miniscan dwell time per pixel (us)"=0.0, "Number of pixels in miniscan"=0.0, "poi dwell time"=0.0, "Rectangle ROI length"=0.0, "Rectangle ROI height"=0.0, "AOL Mode"=enum."Raster", "Plane Mode"=0, "video length (sec)"=0.0, "Frame rate (fps)"=0.0, "Stimuli Timing (usec)"=0.0, "Acquisition Length"=0.0, "Basic Image meta data"={"Wavelength (nm)"=0.0, "# averaged frames"=0.0, "laser power (%)"=0.0, "Pockels"=0.0, "pixel dwell time (us)"=0.0, "pmt 1"=0.0, "pmt 2"=0.0, "back apperture"=0.0, "zoom"=0.0, "field of view"=0.0, "Frame Size"=0, "AOL x centre"=0.0, "AOL y centre"=0.0, "Stage x position"=0.0, "Stage y position"=0.0, "Stage z position"=0.0}, "Z Start (um)"=0.0, "Z Stop (um)"=0.0}, "CALIBRATION"={"Pockels Calibration File"=path "", "Calibration_ini file"=path "", "Setup_ini file"=path ""}, "STATISTICS"={"Z-stack duration (sec)"=0.0, "Number of acquired data-points"=0.0, "Acquisition time (ms)"=0.0, "Number of acquired frames"=0.0, "Intertrial times"=[]}, "BIOLOGY INFORMATION"={"Animal Code or Name"="", "Animal DoB"="", "Animal Age"="", "Animal Sex"="", "Animal Weight"="", "Date of Injection"="", "Date of Implant"="", "Site of Injection"="", "Animal Ear Notch"="", "AAV constructs"="", "Genetic background"="", "Optical reporter"="", "Region of brain imaged"="", "Other \ncomments"=""}} ("All header parameters in"), "IMAGING MODES"=w36) -> (w35:T6)
    }
    frame "TIME SERIES" {
      n22 = global read "General Globals.vi" "Timelapse?"() -> (w40:bool)
      n23 = case shown="True" w40 {
        tunnel: [T6 {"LOGIN"={"User"="Olympus  20X", "Profile"="", "Software Version"="", "Experiment Date Time"=timestamp(0 s since 1904-01-01)}, "GLOBAL PARAMETERS"={"MicroscopeID"="", "Microscope Type"="", "Objective"="", "Field of View (um)"=0.0, "Fill time (us)"=0.0, "Experiment Type"=enum."In vivo", "Stimuli Trigger"=FALSE, "Speed Logging"=FALSE}, "IMAGING MODES"={"Time Series"=FALSE, "Motor Zstack"=FALSE, "AOL Zstack"=FALSE, "Functional Imaging"=FALSE, "Volume Imaging"=FALSE}, "TIME SERIES"={"Basic Image meta data"={"Wavelength (nm)"=0.0, "# averaged frames"=0.0, "laser power (%)"=0.0, "Pockels"=0.0, "pixel dwell time (us)"=0.0, "pmt 1"=0.0, "pmt 2"=0.0, "back apperture"=0.0, "zoom"=0.0, "field of view"=0.0, "Frame Size"=0, "AOL x centre"=0.0, "AOL y centre"=0.0, "Stage x position"=0.0, "Stage y position"=0.0, "Stage z position"=0.0}, "AOL z"=0.0}, "MOTOR Z-STACK "={"Hdr Basic Image meta data"={"Wavelength (nm)"=0.0, "# averaged frames"=0.0, "laser power (%)"=0.0, "Pockels"=0.0, "pixel dwell time (us)"=0.0, "pmt 1"=0.0, "pmt 2"=0.0, "back apperture"=0.0, "zoom"=0.0, "field of view"=0.0, "Frame Size"=0, "AOL x centre"=0.0, "AOL y centre"=0.0, "Stage x position"=0.0, "Stage y position"=0.0, "Stage z position"=0.0}, "Z Start"=0.0, "Z Stop"=0.0, "No of Planes"=0}, "AOL Z-STACK"={"Hdr Basic Image meta data"={"Wavelength (nm)"=0.0, "# averaged frames"=0.0, "laser power (%)"=0.0, "Pockels"=0.0, "pixel dwell time (us)"=0.0, "pmt 1"=0.0, "pmt 2"=0.0, "back apperture"=0.0, "zoom"=0.0, "field of view"=0.0, "Frame Size"=0, "AOL x centre"=0.0, "AOL y centre"=0.0, "Stage x position"=0.0, "Stage y position"=0.0, "Stage z position"=0.0}, "Z Start"=0.0, "Z Stop"=0.0, "No of Planes"=0}, "FUNCTIONAL IMAGING"={"Functional Mode"=enum."Point", "Pockels Modulation"=FALSE, "Number of pois"=0.0, "Number of miniscans"=0.0, "Number of cycles"=0.0, "Number of trials"=0.0, "Miniscan dwell time per pixel (us)"=0.0, "Number of pixels in miniscan"=0.0, "poi dwell time"=0.0, "Rectangle ROI length"=0.0, "Rectangle ROI height"=0.0, "AOL Mode"=enum."Raster", "Plane Mode"=0, "video length (sec)"=0.0, "Frame rate (fps)"=0.0, "Stimuli Timing (usec)"=0.0, "Acquisition Length"=0.0, "Basic Image meta data"={"Wavelength (nm)"=0.0, "# averaged frames"=0.0, "laser power (%)"=0.0, "Pockels"=0.0, "pixel dwell time (us)"=0.0, "pmt 1"=0.0, "pmt 2"=0.0, "back apperture"=0.0, "zoom"=0.0, "field of view"=0.0, "Frame Size"=0, "AOL x centre"=0.0, "AOL y centre"=0.0, "Stage x position"=0.0, "Stage y position"=0.0, "Stage z position"=0.0}, "Z Start (um)"=0.0, "Z Stop (um)"=0.0}, "VOLUME IMAGING"={"Functional Mode"=enum."Point", "Pockels Modulation"=FALSE, "Number of pois"=0.0, "Number of miniscans"=0.0, "Number of cycles"=0.0, "Number of trials"=0.0, "Miniscan dwell time per pixel (us)"=0.0, "Number of pixels in miniscan"=0.0, "poi dwell time"=0.0, "Rectangle ROI length"=0.0, "Rectangle ROI height"=0.0, "AOL Mode"=enum."Raster", "Plane Mode"=0, "video length (sec)"=0.0, "Frame rate (fps)"=0.0, "Stimuli Timing (usec)"=0.0, "Acquisition Length"=0.0, "Basic Image meta data"={"Wavelength (nm)"=0.0, "# averaged frames"=0.0, "laser power (%)"=0.0, "Pockels"=0.0, "pixel dwell time (us)"=0.0, "pmt 1"=0.0, "pmt 2"=0.0, "back apperture"=0.0, "zoom"=0.0, "field of view"=0.0, "Frame Size"=0, "AOL x centre"=0.0, "AOL y centre"=0.0, "Stage x position"=0.0, "Stage y position"=0.0, "Stage z position"=0.0}, "Z Start (um)"=0.0, "Z Stop (um)"=0.0}, "CALIBRATION"={"Pockels Calibration File"=path "", "Calibration_ini file"=path "", "Setup_ini file"=path ""}, "STATISTICS"={"Z-stack duration (sec)"=0.0, "Number of acquired data-points"=0.0, "Acquisition time (ms)"=0.0, "Number of acquired frames"=0.0, "Intertrial times"=[]}, "BIOLOGY INFORMATION"={"Animal Code or Name"="", "Animal DoB"="", "Animal Age"="", "Animal Sex"="", "Animal Weight"="", "Date of Injection"="", "Date of Implant"="", "Site of Injection"="", "Animal Ear Notch"="", "AAV constructs"="", "Genetic background"="", "Optical reporter"="", "Region of brain imaged"="", "Other \ncomments"=""}} ("All header parameters in") w46] -> w42
        tunnel: w41 -> [_ w45]
        frame False {
        }
        frame True {
          n24 = call "Experiment header-bundle basic image meta data.vi"("AOL_Globals"=w45) -> ("Basic image meta-data"=w50:T12)  [unwired: 10 in]
          n25 = Unbundle By Name(w45) -> ("AOL Z"=w44:dbl)
          n26 = Bundle By Name(cluster=T11 {"Basic Image meta data"={"Wavelength (nm)"=0.0, "# averaged frames"=0.0, "laser power (%)"=0.0, "Pockels"=0.0, "pixel dwell time (us)"=0.0, "pmt 1"=0.0, "pmt 2"=0.0, "back apperture"=0.0, "zoom"=0.0, "field of view"=0.0, "Frame Size"=0, "AOL x centre"=0.0, "AOL y centre"=0.0, "Stage x position"=0.0, "Stage y position"=0.0, "Stage z position"=0.0}, "AOL z"=0.0} ("TIME SERIES"), "Basic Image meta data"=w50, "AOL z"=w44) -> (w47:T11)
          n27 = Bundle By Name(cluster=T6 {"LOGIN"={"User"="Olympus  20X", "Profile"="", "Software Version"="", "Experiment Date Time"=timestamp(0 s since 1904-01-01)}, "GLOBAL PARAMETERS"={"MicroscopeID"="", "Microscope Type"="", "Objective"="", "Field of View (um)"=0.0, "Fill time (us)"=0.0, "Experiment Type"=enum."In vivo", "Stimuli Trigger"=FALSE, "Speed Logging"=FALSE}, "IMAGING MODES"={"Time Series"=FALSE, "Motor Zstack"=FALSE, "AOL Zstack"=FALSE, "Functional Imaging"=FALSE, "Volume Imaging"=FALSE}, "TIME SERIES"={"Basic Image meta data"={"Wavelength (nm)"=0.0, "# averaged frames"=0.0, "laser power (%)"=0.0, "Pockels"=0.0, "pixel dwell time (us)"=0.0, "pmt 1"=0.0, "pmt 2"=0.0, "back apperture"=0.0, "zoom"=0.0, "field of view"=0.0, "Frame Size"=0, "AOL x centre"=0.0, "AOL y centre"=0.0, "Stage x position"=0.0, "Stage y position"=0.0, "Stage z position"=0.0}, "AOL z"=0.0}, "MOTOR Z-STACK "={"Hdr Basic Image meta data"={"Wavelength (nm)"=0.0, "# averaged frames"=0.0, "laser power (%)"=0.0, "Pockels"=0.0, "pixel dwell time (us)"=0.0, "pmt 1"=0.0, "pmt 2"=0.0, "back apperture"=0.0, "zoom"=0.0, "field of view"=0.0, "Frame Size"=0, "AOL x centre"=0.0, "AOL y centre"=0.0, "Stage x position"=0.0, "Stage y position"=0.0, "Stage z position"=0.0}, "Z Start"=0.0, "Z Stop"=0.0, "No of Planes"=0}, "AOL Z-STACK"={"Hdr Basic Image meta data"={"Wavelength (nm)"=0.0, "# averaged frames"=0.0, "laser power (%)"=0.0, "Pockels"=0.0, "pixel dwell time (us)"=0.0, "pmt 1"=0.0, "pmt 2"=0.0, "back apperture"=0.0, "zoom"=0.0, "field of view"=0.0, "Frame Size"=0, "AOL x centre"=0.0, "AOL y centre"=0.0, "Stage x position"=0.0, "Stage y position"=0.0, "Stage z position"=0.0}, "Z Start"=0.0, "Z Stop"=0.0, "No of Planes"=0}, "FUNCTIONAL IMAGING"={"Functional Mode"=enum."Point", "Pockels Modulation"=FALSE, "Number of pois"=0.0, "Number of miniscans"=0.0, "Number of cycles"=0.0, "Number of trials"=0.0, "Miniscan dwell time per pixel (us)"=0.0, "Number of pixels in miniscan"=0.0, "poi dwell time"=0.0, "Rectangle ROI length"=0.0, "Rectangle ROI height"=0.0, "AOL Mode"=enum."Raster", "Plane Mode"=0, "video length (sec)"=0.0, "Frame rate (fps)"=0.0, "Stimuli Timing (usec)"=0.0, "Acquisition Length"=0.0, "Basic Image meta data"={"Wavelength (nm)"=0.0, "# averaged frames"=0.0, "laser power (%)"=0.0, "Pockels"=0.0, "pixel dwell time (us)"=0.0, "pmt 1"=0.0, "pmt 2"=0.0, "back apperture"=0.0, "zoom"=0.0, "field of view"=0.0, "Frame Size"=0, "AOL x centre"=0.0, "AOL y centre"=0.0, "Stage x position"=0.0, "Stage y position"=0.0, "Stage z position"=0.0}, "Z Start (um)"=0.0, "Z Stop (um)"=0.0}, "VOLUME IMAGING"={"Functional Mode"=enum."Point", "Pockels Modulation"=FALSE, "Number of pois"=0.0, "Number of miniscans"=0.0, "Number of cycles"=0.0, "Number of trials"=0.0, "Miniscan dwell time per pixel (us)"=0.0, "Number of pixels in miniscan"=0.0, "poi dwell time"=0.0, "Rectangle ROI length"=0.0, "Rectangle ROI height"=0.0, "AOL Mode"=enum."Raster", "Plane Mode"=0, "video length (sec)"=0.0, "Frame rate (fps)"=0.0, "Stimuli Timing (usec)"=0.0, "Acquisition Length"=0.0, "Basic Image meta data"={"Wavelength (nm)"=0.0, "# averaged frames"=0.0, "laser power (%)"=0.0, "Pockels"=0.0, "pixel dwell time (us)"=0.0, "pmt 1"=0.0, "pmt 2"=0.0, "back apperture"=0.0, "zoom"=0.0, "field of view"=0.0, "Frame Size"=0, "AOL x centre"=0.0, "AOL y centre"=0.0, "Stage x position"=0.0, "Stage y position"=0.0, "Stage z position"=0.0}, "Z Start (um)"=0.0, "Z Stop (um)"=0.0}, "CALIBRATION"={"Pockels Calibration File"=path "", "Calibration_ini file"=path "", "Setup_ini file"=path ""}, "STATISTICS"={"Z-stack duration (sec)"=0.0, "Number of acquired data-points"=0.0, "Acquisition time (ms)"=0.0, "Number of acquired frames"=0.0, "Intertrial times"=[]}, "BIOLOGY INFORMATION"={"Animal Code or Name"="", "Animal DoB"="", "Animal Age"="", "Animal Sex"="", "Animal Weight"="", "Date of Injection"="", "Date of Implant"="", "Site of Injection"="", "Animal Ear Notch"="", "AAV constructs"="", "Genetic background"="", "Optical reporter"="", "Region of brain imaged"="", "Other \ncomments"=""}} ("All header parameters in"), "TIME SERIES"=w47) -> (w46:T6)
        }
      }
    }
    frame "MOTOR Z-STACK" {
      n28 = call "Experiment header-bundle basic image meta data.vi"("AOL_Globals"=w54) -> ("Basic image meta-data"=w59:T12)  [unwired: 10 in]
      n29 = Unbundle By Name(w54) -> ("Z Start"=w52:dbl, "Z Stop"=w51:dbl, "# Planes"=w53:i32)
      n30 = Bundle By Name(cluster=T13 {"Hdr Basic Image meta data"={"Wavelength (nm)"=0.0, "# averaged frames"=0.0, "laser power (%)"=0.0, "Pockels"=0.0, "pixel dwell time (us)"=0.0, "pmt 1"=0.0, "pmt 2"=0.0, "back apperture"=0.0, "zoom"=0.0, "field of view"=0.0, "Frame Size"=0, "AOL x centre"=0.0, "AOL y centre"=0.0, "Stage x position"=0.0, "Stage y position"=0.0, "Stage z position"=0.0}, "Z Start"=0.0, "Z Stop"=0.0, "No of Planes"=0} ("MOTOR Z-STACK"), "Hdr Basic Image meta data"=w59, "Z Start"=w52, "Z Stop"=w51, "No of Planes"=w53) -> (w56:T13)
      n31 = Bundle By Name(cluster=T6 {"LOGIN"={"User"="Olympus  20X", "Profile"="", "Software Version"="", "Experiment Date Time"=timestamp(0 s since 1904-01-01)}, "GLOBAL PARAMETERS"={"MicroscopeID"="", "Microscope Type"="", "Objective"="", "Field of View (um)"=0.0, "Fill time (us)"=0.0, "Experiment Type"=enum."In vivo", "Stimuli Trigger"=FALSE, "Speed Logging"=FALSE}, "IMAGING MODES"={"Time Series"=FALSE, "Motor Zstack"=FALSE, "AOL Zstack"=FALSE, "Functional Imaging"=FALSE, "Volume Imaging"=FALSE}, "TIME SERIES"={"Basic Image meta data"={"Wavelength (nm)"=0.0, "# averaged frames"=0.0, "laser power (%)"=0.0, "Pockels"=0.0, "pixel dwell time (us)"=0.0, "pmt 1"=0.0, "pmt 2"=0.0, "back apperture"=0.0, "zoom"=0.0, "field of view"=0.0, "Frame Size"=0, "AOL x centre"=0.0, "AOL y centre"=0.0, "Stage x position"=0.0, "Stage y position"=0.0, "Stage z position"=0.0}, "AOL z"=0.0}, "MOTOR Z-STACK "={"Hdr Basic Image meta data"={"Wavelength (nm)"=0.0, "# averaged frames"=0.0, "laser power (%)"=0.0, "Pockels"=0.0, "pixel dwell time (us)"=0.0, "pmt 1"=0.0, "pmt 2"=0.0, "back apperture"=0.0, "zoom"=0.0, "field of view"=0.0, "Frame Size"=0, "AOL x centre"=0.0, "AOL y centre"=0.0, "Stage x position"=0.0, "Stage y position"=0.0, "Stage z position"=0.0}, "Z Start"=0.0, "Z Stop"=0.0, "No of Planes"=0}, "AOL Z-STACK"={"Hdr Basic Image meta data"={"Wavelength (nm)"=0.0, "# averaged frames"=0.0, "laser power (%)"=0.0, "Pockels"=0.0, "pixel dwell time (us)"=0.0, "pmt 1"=0.0, "pmt 2"=0.0, "back apperture"=0.0, "zoom"=0.0, "field of view"=0.0, "Frame Size"=0, "AOL x centre"=0.0, "AOL y centre"=0.0, "Stage x position"=0.0, "Stage y position"=0.0, "Stage z position"=0.0}, "Z Start"=0.0, "Z Stop"=0.0, "No of Planes"=0}, "FUNCTIONAL IMAGING"={"Functional Mode"=enum."Point", "Pockels Modulation"=FALSE, "Number of pois"=0.0, "Number of miniscans"=0.0, "Number of cycles"=0.0, "Number of trials"=0.0, "Miniscan dwell time per pixel (us)"=0.0, "Number of pixels in miniscan"=0.0, "poi dwell time"=0.0, "Rectangle ROI length"=0.0, "Rectangle ROI height"=0.0, "AOL Mode"=enum."Raster", "Plane Mode"=0, "video length (sec)"=0.0, "Frame rate (fps)"=0.0, "Stimuli Timing (usec)"=0.0, "Acquisition Length"=0.0, "Basic Image meta data"={"Wavelength (nm)"=0.0, "# averaged frames"=0.0, "laser power (%)"=0.0, "Pockels"=0.0, "pixel dwell time (us)"=0.0, "pmt 1"=0.0, "pmt 2"=0.0, "back apperture"=0.0, "zoom"=0.0, "field of view"=0.0, "Frame Size"=0, "AOL x centre"=0.0, "AOL y centre"=0.0, "Stage x position"=0.0, "Stage y position"=0.0, "Stage z position"=0.0}, "Z Start (um)"=0.0, "Z Stop (um)"=0.0}, "VOLUME IMAGING"={"Functional Mode"=enum."Point", "Pockels Modulation"=FALSE, "Number of pois"=0.0, "Number of miniscans"=0.0, "Number of cycles"=0.0, "Number of trials"=0.0, "Miniscan dwell time per pixel (us)"=0.0, "Number of pixels in miniscan"=0.0, "poi dwell time"=0.0, "Rectangle ROI length"=0.0, "Rectangle ROI height"=0.0, "AOL Mode"=enum."Raster", "Plane Mode"=0, "video length (sec)"=0.0, "Frame rate (fps)"=0.0, "Stimuli Timing (usec)"=0.0, "Acquisition Length"=0.0, "Basic Image meta data"={"Wavelength (nm)"=0.0, "# averaged frames"=0.0, "laser power (%)"=0.0, "Pockels"=0.0, "pixel dwell time (us)"=0.0, "pmt 1"=0.0, "pmt 2"=0.0, "back apperture"=0.0, "zoom"=0.0, "field of view"=0.0, "Frame Size"=0, "AOL x centre"=0.0, "AOL y centre"=0.0, "Stage x position"=0.0, "Stage y position"=0.0, "Stage z position"=0.0}, "Z Start (um)"=0.0, "Z Stop (um)"=0.0}, "CALIBRATION"={"Pockels Calibration File"=path "", "Calibration_ini file"=path "", "Setup_ini file"=path ""}, "STATISTICS"={"Z-stack duration (sec)"=0.0, "Number of acquired data-points"=0.0, "Acquisition time (ms)"=0.0, "Number of acquired frames"=0.0, "Intertrial times"=[]}, "BIOLOGY INFORMATION"={"Animal Code or Name"="", "Animal DoB"="", "Animal Age"="", "Animal Sex"="", "Animal Weight"="", "Date of Injection"="", "Date of Implant"="", "Site of Injection"="", "Animal Ear Notch"="", "AAV constructs"="", "Genetic background"="", "Optical reporter"="", "Region of brain imaged"="", "Other \ncomments"=""}} ("All header parameters in"), "MOTOR Z-STACK"=w56) -> (w55:T6)
    }
    frame "AOL Z-STACK" {
      n32 = call "Experiment header-bundle basic image meta data.vi"("AOL_Globals"=w63) -> ("Basic image meta-data"=w68:T12)  [unwired: 10 in]
      n33 = Unbundle By Name(w63) -> ("Z Start"=w62:dbl, "Z Stop"=w61:dbl, "# Planes"=w60:i32)
      n34 = Bundle By Name(cluster=T14 {"Hdr Basic Image meta data"={"Wavelength (nm)"=0.0, "# averaged frames"=0.0, "laser power (%)"=0.0, "Pockels"=0.0, "pixel dwell time (us)"=0.0, "pmt 1"=0.0, "pmt 2"=0.0, "back apperture"=0.0, "zoom"=0.0, "field of view"=0.0, "Frame Size"=0, "AOL x centre"=0.0, "AOL y centre"=0.0, "Stage x position"=0.0, "Stage y position"=0.0, "Stage z position"=0.0}, "Z Start"=0.0, "Z Stop"=0.0, "No of Planes"=0} ("AOL Z-STACK"), "Hdr Basic Image meta data"=w68, "Z Start"=w62, "Z Stop"=w61, "No of Planes"=w60) -> (w67:T14)
      n35 = Bundle By Name(cluster=T6 {"LOGIN"={"User"="Olympus  20X", "Profile"="", "Software Version"="", "Experiment Date Time"=timestamp(0 s since 1904-01-01)}, "GLOBAL PARAMETERS"={"MicroscopeID"="", "Microscope Type"="", "Objective"="", "Field of View (um)"=0.0, "Fill time (us)"=0.0, "Experiment Type"=enum."In vivo", "Stimuli Trigger"=FALSE, "Speed Logging"=FALSE}, "IMAGING MODES"={"Time Series"=FALSE, "Motor Zstack"=FALSE, "AOL Zstack"=FALSE, "Functional Imaging"=FALSE, "Volume Imaging"=FALSE}, "TIME SERIES"={"Basic Image meta data"={"Wavelength (nm)"=0.0, "# averaged frames"=0.0, "laser power (%)"=0.0, "Pockels"=0.0, "pixel dwell time (us)"=0.0, "pmt 1"=0.0, "pmt 2"=0.0, "back apperture"=0.0, "zoom"=0.0, "field of view"=0.0, "Frame Size"=0, "AOL x centre"=0.0, "AOL y centre"=0.0, "Stage x position"=0.0, "Stage y position"=0.0, "Stage z position"=0.0}, "AOL z"=0.0}, "MOTOR Z-STACK "={"Hdr Basic Image meta data"={"Wavelength (nm)"=0.0, "# averaged frames"=0.0, "laser power (%)"=0.0, "Pockels"=0.0, "pixel dwell time (us)"=0.0, "pmt 1"=0.0, "pmt 2"=0.0, "back apperture"=0.0, "zoom"=0.0, "field of view"=0.0, "Frame Size"=0, "AOL x centre"=0.0, "AOL y centre"=0.0, "Stage x position"=0.0, "Stage y position"=0.0, "Stage z position"=0.0}, "Z Start"=0.0, "Z Stop"=0.0, "No of Planes"=0}, "AOL Z-STACK"={"Hdr Basic Image meta data"={"Wavelength (nm)"=0.0, "# averaged frames"=0.0, "laser power (%)"=0.0, "Pockels"=0.0, "pixel dwell time (us)"=0.0, "pmt 1"=0.0, "pmt 2"=0.0, "back apperture"=0.0, "zoom"=0.0, "field of view"=0.0, "Frame Size"=0, "AOL x centre"=0.0, "AOL y centre"=0.0, "Stage x position"=0.0, "Stage y position"=0.0, "Stage z position"=0.0}, "Z Start"=0.0, "Z Stop"=0.0, "No of Planes"=0}, "FUNCTIONAL IMAGING"={"Functional Mode"=enum."Point", "Pockels Modulation"=FALSE, "Number of pois"=0.0, "Number of miniscans"=0.0, "Number of cycles"=0.0, "Number of trials"=0.0, "Miniscan dwell time per pixel (us)"=0.0, "Number of pixels in miniscan"=0.0, "poi dwell time"=0.0, "Rectangle ROI length"=0.0, "Rectangle ROI height"=0.0, "AOL Mode"=enum."Raster", "Plane Mode"=0, "video length (sec)"=0.0, "Frame rate (fps)"=0.0, "Stimuli Timing (usec)"=0.0, "Acquisition Length"=0.0, "Basic Image meta data"={"Wavelength (nm)"=0.0, "# averaged frames"=0.0, "laser power (%)"=0.0, "Pockels"=0.0, "pixel dwell time (us)"=0.0, "pmt 1"=0.0, "pmt 2"=0.0, "back apperture"=0.0, "zoom"=0.0, "field of view"=0.0, "Frame Size"=0, "AOL x centre"=0.0, "AOL y centre"=0.0, "Stage x position"=0.0, "Stage y position"=0.0, "Stage z position"=0.0}, "Z Start (um)"=0.0, "Z Stop (um)"=0.0}, "VOLUME IMAGING"={"Functional Mode"=enum."Point", "Pockels Modulation"=FALSE, "Number of pois"=0.0, "Number of miniscans"=0.0, "Number of cycles"=0.0, "Number of trials"=0.0, "Miniscan dwell time per pixel (us)"=0.0, "Number of pixels in miniscan"=0.0, "poi dwell time"=0.0, "Rectangle ROI length"=0.0, "Rectangle ROI height"=0.0, "AOL Mode"=enum."Raster", "Plane Mode"=0, "video length (sec)"=0.0, "Frame rate (fps)"=0.0, "Stimuli Timing (usec)"=0.0, "Acquisition Length"=0.0, "Basic Image meta data"={"Wavelength (nm)"=0.0, "# averaged frames"=0.0, "laser power (%)"=0.0, "Pockels"=0.0, "pixel dwell time (us)"=0.0, "pmt 1"=0.0, "pmt 2"=0.0, "back apperture"=0.0, "zoom"=0.0, "field of view"=0.0, "Frame Size"=0, "AOL x centre"=0.0, "AOL y centre"=0.0, "Stage x position"=0.0, "Stage y position"=0.0, "Stage z position"=0.0}, "Z Start (um)"=0.0, "Z Stop (um)"=0.0}, "CALIBRATION"={"Pockels Calibration File"=path "", "Calibration_ini file"=path "", "Setup_ini file"=path ""}, "STATISTICS"={"Z-stack duration (sec)"=0.0, "Number of acquired data-points"=0.0, "Acquisition time (ms)"=0.0, "Number of acquired frames"=0.0, "Intertrial times"=[]}, "BIOLOGY INFORMATION"={"Animal Code or Name"="", "Animal DoB"="", "Animal Age"="", "Animal Sex"="", "Animal Weight"="", "Date of Injection"="", "Date of Implant"="", "Site of Injection"="", "Animal Ear Notch"="", "AAV constructs"="", "Genetic background"="", "Optical reporter"="", "Region of brain imaged"="", "Other \ncomments"=""}} ("All header parameters in"), "AOL Z-STACK"=w67) -> (w66:T6)
    }
    frame "FUNCTIONAL IMAGING" {
      n36 = Unbundle By Name(w71) -> ("Functional Mode"=w91:T16, "Number of POI"=w89:u16, "Number of Miniscans"=w88:u16, "Number of Cycles"=w87:u64, "Number of Trials"=w86:u16, "Miniscan Dwell time per pixel (us)"=w85:dbl, "Number of Pixels in Miniscan"=w84:u16, "POI Dwell time (us)"=w83:dbl, "Rectangle ROI length (pixels)"=w82:u16, "Rectangle ROI height (pixels)"=w81:u16, "AOL Mode"=w80:T17, "Plane Mode"=w79:T18, "Acquisition Length (sec)"=w78:dbl)
      n37 = global read "gl_Pockels control globals.vi" "Funct. acq. pockels modulation?"() -> (w90:bool)
      n38 = call "Experiment header-Calculate frame rate.vi"("AOL_Globals"=w71) -> ("FrameRate (fps)"=w76:dbl)  [unwired: 10 in]
      n39 = call "fgv_StimTrigLive-Setup.vi"("Function"=enum16{"Intialize", "Write", "Read", "Clear"}."Read") -> ("Live stim.trig.period (sec)"=w74:dbl)  [unwired: 11 in, 3 out]
      n40 = call "Experiment header-bundle basic image meta data.vi"("AOL_Globals"=w71) -> ("Basic image meta-data"=w95:T12)  [unwired: 10 in]
      n41 = Unbundle By Name(w71) -> ("Z Start"=w70:dbl, "Z Stop"=w69:dbl)
      n42 = Multiply(x=w74, y=1000.0 ("x")) -> (x*y=w72:dbl)
      n43 = Bundle By Name(cluster=T15 {"Functional Mode"=enum."Point", "Pockels Modulation"=FALSE, "Number of pois"=0.0, "Number of miniscans"=0.0, "Number of cycles"=0.0, "Number of trials"=0.0, "Miniscan dwell time per pixel (us)"=0.0, "Number of pixels in miniscan"=0.0, "poi dwell time"=0.0, "Rectangle ROI length"=0.0, "Rectangle ROI height"=0.0, "AOL Mode"=enum."Raster", "Plane Mode"=0, "video length (sec)"=0.0, "Frame rate (fps)"=0.0, "Stimuli Timing (usec)"=0.0, "Acquisition Length"=0.0, "Basic Image meta data"={"Wavelength (nm)"=0.0, "# averaged frames"=0.0, "laser power (%)"=0.0, "Pockels"=0.0, "pixel dwell time (us)"=0.0, "pmt 1"=0.0, "pmt 2"=0.0, "back apperture"=0.0, "zoom"=0.0, "field of view"=0.0, "Frame Size"=0, "AOL x centre"=0.0, "AOL y centre"=0.0, "Stage x position"=0.0, "Stage y position"=0.0, "Stage z position"=0.0}, "Z Start (um)"=0.0, "Z Stop (um)"=0.0} ("FUNCTIONAL IMAGING"), "Pockels Modulation"=w90, "Functional Mode"=w91, "Number of pois"=w89, "Number of miniscans"=w88, "Number of cycles"=w87, "Number of trials"=w86, "Miniscan dwell time per pixel (us)"=w85, "Number of pixels in miniscan"=w84, "poi dwell time"=w83, "Rectangle ROI length"=w82, "Rectangle ROI height"=w81, "AOL Mode"=w80, "Plane Mode"=w79, "Acquisition Length"=w78, "Frame rate (fps)"=w76, "Stimuli Timing (usec)"=w72, "video length (sec)"=0.0, "Basic Image meta data"=w95, "Z Start (um)"=w70, "Z Stop (um)"=w69) -> (w92:T15)
      n44 = Bundle By Name(cluster=T6 {"LOGIN"={"User"="Olympus  20X", "Profile"="", "Software Version"="", "Experiment Date Time"=timestamp(0 s since 1904-01-01)}, "GLOBAL PARAMETERS"={"MicroscopeID"="", "Microscope Type"="", "Objective"="", "Field of View (um)"=0.0, "Fill time (us)"=0.0, "Experiment Type"=enum."In vivo", "Stimuli Trigger"=FALSE, "Speed Logging"=FALSE}, "IMAGING MODES"={"Time Series"=FALSE, "Motor Zstack"=FALSE, "AOL Zstack"=FALSE, "Functional Imaging"=FALSE, "Volume Imaging"=FALSE}, "TIME SERIES"={"Basic Image meta data"={"Wavelength (nm)"=0.0, "# averaged frames"=0.0, "laser power (%)"=0.0, "Pockels"=0.0, "pixel dwell time (us)"=0.0, "pmt 1"=0.0, "pmt 2"=0.0, "back apperture"=0.0, "zoom"=0.0, "field of view"=0.0, "Frame Size"=0, "AOL x centre"=0.0, "AOL y centre"=0.0, "Stage x position"=0.0, "Stage y position"=0.0, "Stage z position"=0.0}, "AOL z"=0.0}, "MOTOR Z-STACK "={"Hdr Basic Image meta data"={"Wavelength (nm)"=0.0, "# averaged frames"=0.0, "laser power (%)"=0.0, "Pockels"=0.0, "pixel dwell time (us)"=0.0, "pmt 1"=0.0, "pmt 2"=0.0, "back apperture"=0.0, "zoom"=0.0, "field of view"=0.0, "Frame Size"=0, "AOL x centre"=0.0, "AOL y centre"=0.0, "Stage x position"=0.0, "Stage y position"=0.0, "Stage z position"=0.0}, "Z Start"=0.0, "Z Stop"=0.0, "No of Planes"=0}, "AOL Z-STACK"={"Hdr Basic Image meta data"={"Wavelength (nm)"=0.0, "# averaged frames"=0.0, "laser power (%)"=0.0, "Pockels"=0.0, "pixel dwell time (us)"=0.0, "pmt 1"=0.0, "pmt 2"=0.0, "back apperture"=0.0, "zoom"=0.0, "field of view"=0.0, "Frame Size"=0, "AOL x centre"=0.0, "AOL y centre"=0.0, "Stage x position"=0.0, "Stage y position"=0.0, "Stage z position"=0.0}, "Z Start"=0.0, "Z Stop"=0.0, "No of Planes"=0}, "FUNCTIONAL IMAGING"={"Functional Mode"=enum."Point", "Pockels Modulation"=FALSE, "Number of pois"=0.0, "Number of miniscans"=0.0, "Number of cycles"=0.0, "Number of trials"=0.0, "Miniscan dwell time per pixel (us)"=0.0, "Number of pixels in miniscan"=0.0, "poi dwell time"=0.0, "Rectangle ROI length"=0.0, "Rectangle ROI height"=0.0, "AOL Mode"=enum."Raster", "Plane Mode"=0, "video length (sec)"=0.0, "Frame rate (fps)"=0.0, "Stimuli Timing (usec)"=0.0, "Acquisition Length"=0.0, "Basic Image meta data"={"Wavelength (nm)"=0.0, "# averaged frames"=0.0, "laser power (%)"=0.0, "Pockels"=0.0, "pixel dwell time (us)"=0.0, "pmt 1"=0.0, "pmt 2"=0.0, "back apperture"=0.0, "zoom"=0.0, "field of view"=0.0, "Frame Size"=0, "AOL x centre"=0.0, "AOL y centre"=0.0, "Stage x position"=0.0, "Stage y position"=0.0, "Stage z position"=0.0}, "Z Start (um)"=0.0, "Z Stop (um)"=0.0}, "VOLUME IMAGING"={"Functional Mode"=enum."Point", "Pockels Modulation"=FALSE, "Number of pois"=0.0, "Number of miniscans"=0.0, "Number of cycles"=0.0, "Number of trials"=0.0, "Miniscan dwell time per pixel (us)"=0.0, "Number of pixels in miniscan"=0.0, "poi dwell time"=0.0, "Rectangle ROI length"=0.0, "Rectangle ROI height"=0.0, "AOL Mode"=enum."Raster", "Plane Mode"=0, "video length (sec)"=0.0, "Frame rate (fps)"=0.0, "Stimuli Timing (usec)"=0.0, "Acquisition Length"=0.0, "Basic Image meta data"={"Wavelength (nm)"=0.0, "# averaged frames"=0.0, "laser power (%)"=0.0, "Pockels"=0.0, "pixel dwell time (us)"=0.0, "pmt 1"=0.0, "pmt 2"=0.0, "back apperture"=0.0, "zoom"=0.0, "field of view"=0.0, "Frame Size"=0, "AOL x centre"=0.0, "AOL y centre"=0.0, "Stage x position"=0.0, "Stage y position"=0.0, "Stage z position"=0.0}, "Z Start (um)"=0.0, "Z Stop (um)"=0.0}, "CALIBRATION"={"Pockels Calibration File"=path "", "Calibration_ini file"=path "", "Setup_ini file"=path ""}, "STATISTICS"={"Z-stack duration (sec)"=0.0, "Number of acquired data-points"=0.0, "Acquisition time (ms)"=0.0, "Number of acquired frames"=0.0, "Intertrial times"=[]}, "BIOLOGY INFORMATION"={"Animal Code or Name"="", "Animal DoB"="", "Animal Age"="", "Animal Sex"="", "Animal Weight"="", "Date of Injection"="", "Date of Implant"="", "Site of Injection"="", "Animal Ear Notch"="", "AAV constructs"="", "Genetic background"="", "Optical reporter"="", "Region of brain imaged"="", "Other \ncomments"=""}} ("All header parameters in"), "FUNCTIONAL IMAGING"=w92) -> (w93:T6)
    }
    frame "VOLUME IMAGING" {
      n45 = Unbundle By Name(w100) -> ("Functional Mode"=w120:T16, "Number of POI"=w118:u16, "Number of Miniscans"=w117:u16, "Number of Cycles"=w116:u64, "Number of Trials"=w115:u16, "Miniscan Dwell time per pixel (us)"=w114:dbl, "Number of Pixels in Miniscan"=w113:u16, "POI Dwell time (us)"=w112:dbl, "Rectangle ROI length (pixels)"=w111:u16, "Rectangle ROI height (pixels)"=w110:u16, "AOL Mode"=w109:T17, "Plane Mode"=w108:T18, "Acquisition Length (sec)"=w107:dbl)
      n46 = global read "gl_Pockels control globals.vi" "Funct. acq. pockels modulation?"() -> (w119:bool)
      n47 = call "Experiment header-Calculate frame rate.vi"("AOL_Globals"=w100) -> ("FrameRate (fps)"=w105:dbl)  [unwired: 10 in]
      n48 = call "fgv_StimTrigLive-Setup.vi"("Function"=enum16{"Intialize", "Write", "Read", "Clear"}."Read") -> ("Live stim.trig.period (sec)"=w103:dbl)  [unwired: 11 in, 3 out]
      n49 = call "Experiment header-bundle basic image meta data.vi"("AOL_Globals"=w100) -> ("Basic image meta-data"=w124:T12)  [unwired: 10 in]
      n50 = Unbundle By Name(w100) -> ("Z Start"=w99:dbl, "Z Stop"=w98:dbl)
      n51 = Multiply(x=w103, y=1000.0 ("x")) -> (x*y=w101:dbl)
      n52 = Bundle By Name(cluster=T23 {"Functional Mode"=enum."Point", "Pockels Modulation"=FALSE, "Number of pois"=0.0, "Number of miniscans"=0.0, "Number of cycles"=0.0, "Number of trials"=0.0, "Miniscan dwell time per pixel (us)"=0.0, "Number of pixels in miniscan"=0.0, "poi dwell time"=0.0, "Rectangle ROI length"=0.0, "Rectangle ROI height"=0.0, "AOL Mode"=enum."Raster", "Plane Mode"=0, "video length (sec)"=0.0, "Frame rate (fps)"=0.0, "Stimuli Timing (usec)"=0.0, "Acquisition Length"=0.0, "Basic Image meta data"={"Wavelength (nm)"=0.0, "# averaged frames"=0.0, "laser power (%)"=0.0, "Pockels"=0.0, "pixel dwell time (us)"=0.0, "pmt 1"=0.0, "pmt 2"=0.0, "back apperture"=0.0, "zoom"=0.0, "field of view"=0.0, "Frame Size"=0, "AOL x centre"=0.0, "AOL y centre"=0.0, "Stage x position"=0.0, "Stage y position"=0.0, "Stage z position"=0.0}, "Z Start (um)"=0.0, "Z Stop (um)"=0.0} ("FUNCTIONAL IMAGING"), "Pockels Modulation"=w119, "Functional Mode"=w120, "Number of pois"=w118, "Number of miniscans"=w117, "Number of cycles"=w116, "Number of trials"=w115, "Miniscan dwell time per pixel (us)"=w114, "Number of pixels in miniscan"=w113, "poi dwell time"=w112, "Rectangle ROI length"=w111, "Rectangle ROI height"=w110, "AOL Mode"=w109, "Plane Mode"=w108, "Acquisition Length"=w107, "Frame rate (fps)"=w105, "Stimuli Timing (usec)"=w101, "video length (sec)"=0.0, "Basic Image meta data"=w124, "Z Start (um)"=w99, "Z Stop (um)"=w98) -> (w121:T23)
      n53 = Bundle By Name(cluster=T6 {"LOGIN"={"User"="Olympus  20X", "Profile"="", "Software Version"="", "Experiment Date Time"=timestamp(0 s since 1904-01-01)}, "GLOBAL PARAMETERS"={"MicroscopeID"="", "Microscope Type"="", "Objective"="", "Field of View (um)"=0.0, "Fill time (us)"=0.0, "Experiment Type"=enum."In vivo", "Stimuli Trigger"=FALSE, "Speed Logging"=FALSE}, "IMAGING MODES"={"Time Series"=FALSE, "Motor Zstack"=FALSE, "AOL Zstack"=FALSE, "Functional Imaging"=FALSE, "Volume Imaging"=FALSE}, "TIME SERIES"={"Basic Image meta data"={"Wavelength (nm)"=0.0, "# averaged frames"=0.0, "laser power (%)"=0.0, "Pockels"=0.0, "pixel dwell time (us)"=0.0, "pmt 1"=0.0, "pmt 2"=0.0, "back apperture"=0.0, "zoom"=0.0, "field of view"=0.0, "Frame Size"=0, "AOL x centre"=0.0, "AOL y centre"=0.0, "Stage x position"=0.0, "Stage y position"=0.0, "Stage z position"=0.0}, "AOL z"=0.0}, "MOTOR Z-STACK "={"Hdr Basic Image meta data"={"Wavelength (nm)"=0.0, "# averaged frames"=0.0, "laser power (%)"=0.0, "Pockels"=0.0, "pixel dwell time (us)"=0.0, "pmt 1"=0.0, "pmt 2"=0.0, "back apperture"=0.0, "zoom"=0.0, "field of view"=0.0, "Frame Size"=0, "AOL x centre"=0.0, "AOL y centre"=0.0, "Stage x position"=0.0, "Stage y position"=0.0, "Stage z position"=0.0}, "Z Start"=0.0, "Z Stop"=0.0, "No of Planes"=0}, "AOL Z-STACK"={"Hdr Basic Image meta data"={"Wavelength (nm)"=0.0, "# averaged frames"=0.0, "laser power (%)"=0.0, "Pockels"=0.0, "pixel dwell time (us)"=0.0, "pmt 1"=0.0, "pmt 2"=0.0, "back apperture"=0.0, "zoom"=0.0, "field of view"=0.0, "Frame Size"=0, "AOL x centre"=0.0, "AOL y centre"=0.0, "Stage x position"=0.0, "Stage y position"=0.0, "Stage z position"=0.0}, "Z Start"=0.0, "Z Stop"=0.0, "No of Planes"=0}, "FUNCTIONAL IMAGING"={"Functional Mode"=enum."Point", "Pockels Modulation"=FALSE, "Number of pois"=0.0, "Number of miniscans"=0.0, "Number of cycles"=0.0, "Number of trials"=0.0, "Miniscan dwell time per pixel (us)"=0.0, "Number of pixels in miniscan"=0.0, "poi dwell time"=0.0, "Rectangle ROI length"=0.0, "Rectangle ROI height"=0.0, "AOL Mode"=enum."Raster", "Plane Mode"=0, "video length (sec)"=0.0, "Frame rate (fps)"=0.0, "Stimuli Timing (usec)"=0.0, "Acquisition Length"=0.0, "Basic Image meta data"={"Wavelength (nm)"=0.0, "# averaged frames"=0.0, "laser power (%)"=0.0, "Pockels"=0.0, "pixel dwell time (us)"=0.0, "pmt 1"=0.0, "pmt 2"=0.0, "back apperture"=0.0, "zoom"=0.0, "field of view"=0.0, "Frame Size"=0, "AOL x centre"=0.0, "AOL y centre"=0.0, "Stage x position"=0.0, "Stage y position"=0.0, "Stage z position"=0.0}, "Z Start (um)"=0.0, "Z Stop (um)"=0.0}, "VOLUME IMAGING"={"Functional Mode"=enum."Point", "Pockels Modulation"=FALSE, "Number of pois"=0.0, "Number of miniscans"=0.0, "Number of cycles"=0.0, "Number of trials"=0.0, "Miniscan dwell time per pixel (us)"=0.0, "Number of pixels in miniscan"=0.0, "poi dwell time"=0.0, "Rectangle ROI length"=0.0, "Rectangle ROI height"=0.0, "AOL Mode"=enum."Raster", "Plane Mode"=0, "video length (sec)"=0.0, "Frame rate (fps)"=0.0, "Stimuli Timing (usec)"=0.0, "Acquisition Length"=0.0, "Basic Image meta data"={"Wavelength (nm)"=0.0, "# averaged frames"=0.0, "laser power (%)"=0.0, "Pockels"=0.0, "pixel dwell time (us)"=0.0, "pmt 1"=0.0, "pmt 2"=0.0, "back apperture"=0.0, "zoom"=0.0, "field of view"=0.0, "Frame Size"=0, "AOL x centre"=0.0, "AOL y centre"=0.0, "Stage x position"=0.0, "Stage y position"=0.0, "Stage z position"=0.0}, "Z Start (um)"=0.0, "Z Stop (um)"=0.0}, "CALIBRATION"={"Pockels Calibration File"=path "", "Calibration_ini file"=path "", "Setup_ini file"=path ""}, "STATISTICS"={"Z-stack duration (sec)"=0.0, "Number of acquired data-points"=0.0, "Acquisition time (ms)"=0.0, "Number of acquired frames"=0.0, "Intertrial times"=[]}, "BIOLOGY INFORMATION"={"Animal Code or Name"="", "Animal DoB"="", "Animal Age"="", "Animal Sex"="", "Animal Weight"="", "Date of Injection"="", "Date of Implant"="", "Site of Injection"="", "Animal Ear Notch"="", "AAV constructs"="", "Genetic background"="", "Optical reporter"="", "Region of brain imaged"="", "Other \ncomments"=""}} ("All header parameters in"), "VOLUME IMAGING"=w121) -> (w122:T6)
    }
    frame "CALIBRATION" {
      n54 = global read "gl_Calibration globals.vi" "Pockels cal file name"() -> (w132:string)
      n55 = global read "General Globals.vi" "Config Files Folder Path"() -> (w130:path)
      n56 = Concatenate Strings("Calibration Files\\", w132) -> (w131:string)
      n57 = Build Path(base path=w130, name or relative path=w131) -> (appended path=w128:path)
      n58 = Build Path(base path=w130, name or relative path="Calibration.ini") -> (appended path=w129:path)
      n59 = Build Path(base path=w130, name or relative path="Setup.ini") -> (appended path=w135:path)
      n60 = Bundle By Name(cluster=T19 {"Pockels Calibration File"=path "", "Calibration_ini file"=path "", "Setup_ini file"=path ""} ("CALIBRATION"), "Pockels Calibration File"=w128, "Calibration_ini file"=w129, "Setup_ini file"=w135) -> (w126:T19)
      n61 = Bundle By Name(cluster=T6 {"LOGIN"={"User"="Olympus  20X", "Profile"="", "Software Version"="", "Experiment Date Time"=timestamp(0 s since 1904-01-01)}, "GLOBAL PARAMETERS"={"MicroscopeID"="", "Microscope Type"="", "Objective"="", "Field of View (um)"=0.0, "Fill time (us)"=0.0, "Experiment Type"=enum."In vivo", "Stimuli Trigger"=FALSE, "Speed Logging"=FALSE}, "IMAGING MODES"={"Time Series"=FALSE, "Motor Zstack"=FALSE, "AOL Zstack"=FALSE, "Functional Imaging"=FALSE, "Volume Imaging"=FALSE}, "TIME SERIES"={"Basic Image meta data"={"Wavelength (nm)"=0.0, "# averaged frames"=0.0, "laser power (%)"=0.0, "Pockels"=0.0, "pixel dwell time (us)"=0.0, "pmt 1"=0.0, "pmt 2"=0.0, "back apperture"=0.0, "zoom"=0.0, "field of view"=0.0, "Frame Size"=0, "AOL x centre"=0.0, "AOL y centre"=0.0, "Stage x position"=0.0, "Stage y position"=0.0, "Stage z position"=0.0}, "AOL z"=0.0}, "MOTOR Z-STACK "={"Hdr Basic Image meta data"={"Wavelength (nm)"=0.0, "# averaged frames"=0.0, "laser power (%)"=0.0, "Pockels"=0.0, "pixel dwell time (us)"=0.0, "pmt 1"=0.0, "pmt 2"=0.0, "back apperture"=0.0, "zoom"=0.0, "field of view"=0.0, "Frame Size"=0, "AOL x centre"=0.0, "AOL y centre"=0.0, "Stage x position"=0.0, "Stage y position"=0.0, "Stage z position"=0.0}, "Z Start"=0.0, "Z Stop"=0.0, "No of Planes"=0}, "AOL Z-STACK"={"Hdr Basic Image meta data"={"Wavelength (nm)"=0.0, "# averaged frames"=0.0, "laser power (%)"=0.0, "Pockels"=0.0, "pixel dwell time (us)"=0.0, "pmt 1"=0.0, "pmt 2"=0.0, "back apperture"=0.0, "zoom"=0.0, "field of view"=0.0, "Frame Size"=0, "AOL x centre"=0.0, "AOL y centre"=0.0, "Stage x position"=0.0, "Stage y position"=0.0, "Stage z position"=0.0}, "Z Start"=0.0, "Z Stop"=0.0, "No of Planes"=0}, "FUNCTIONAL IMAGING"={"Functional Mode"=enum."Point", "Pockels Modulation"=FALSE, "Number of pois"=0.0, "Number of miniscans"=0.0, "Number of cycles"=0.0, "Number of trials"=0.0, "Miniscan dwell time per pixel (us)"=0.0, "Number of pixels in miniscan"=0.0, "poi dwell time"=0.0, "Rectangle ROI length"=0.0, "Rectangle ROI height"=0.0, "AOL Mode"=enum."Raster", "Plane Mode"=0, "video length (sec)"=0.0, "Frame rate (fps)"=0.0, "Stimuli Timing (usec)"=0.0, "Acquisition Length"=0.0, "Basic Image meta data"={"Wavelength (nm)"=0.0, "# averaged frames"=0.0, "laser power (%)"=0.0, "Pockels"=0.0, "pixel dwell time (us)"=0.0, "pmt 1"=0.0, "pmt 2"=0.0, "back apperture"=0.0, "zoom"=0.0, "field of view"=0.0, "Frame Size"=0, "AOL x centre"=0.0, "AOL y centre"=0.0, "Stage x position"=0.0, "Stage y position"=0.0, "Stage z position"=0.0}, "Z Start (um)"=0.0, "Z Stop (um)"=0.0}, "VOLUME IMAGING"={"Functional Mode"=enum."Point", "Pockels Modulation"=FALSE, "Number of pois"=0.0, "Number of miniscans"=0.0, "Number of cycles"=0.0, "Number of trials"=0.0, "Miniscan dwell time per pixel (us)"=0.0, "Number of pixels in miniscan"=0.0, "poi dwell time"=0.0, "Rectangle ROI length"=0.0, "Rectangle ROI height"=0.0, "AOL Mode"=enum."Raster", "Plane Mode"=0, "video length (sec)"=0.0, "Frame rate (fps)"=0.0, "Stimuli Timing (usec)"=0.0, "Acquisition Length"=0.0, "Basic Image meta data"={"Wavelength (nm)"=0.0, "# averaged frames"=0.0, "laser power (%)"=0.0, "Pockels"=0.0, "pixel dwell time (us)"=0.0, "pmt 1"=0.0, "pmt 2"=0.0, "back apperture"=0.0, "zoom"=0.0, "field of view"=0.0, "Frame Size"=0, "AOL x centre"=0.0, "AOL y centre"=0.0, "Stage x position"=0.0, "Stage y position"=0.0, "Stage z position"=0.0}, "Z Start (um)"=0.0, "Z Stop (um)"=0.0}, "CALIBRATION"={"Pockels Calibration File"=path "", "Calibration_ini file"=path "", "Setup_ini file"=path ""}, "STATISTICS"={"Z-stack duration (sec)"=0.0, "Number of acquired data-points"=0.0, "Acquisition time (ms)"=0.0, "Number of acquired frames"=0.0, "Intertrial times"=[]}, "BIOLOGY INFORMATION"={"Animal Code or Name"="", "Animal DoB"="", "Animal Age"="", "Animal Sex"="", "Animal Weight"="", "Date of Injection"="", "Date of Implant"="", "Site of Injection"="", "Animal Ear Notch"="", "AAV constructs"="", "Genetic background"="", "Optical reporter"="", "Region of brain imaged"="", "Other \ncomments"=""}} ("All header parameters in"), "CALIBRATION"=w126) -> (w125:T6)
    }
    frame "STATISTICS" {
      # "THE VALUES ARE CORRECT ONLY WHEN CALLED AFTER THE LAST\nTRIAL OR WHEN FUNCTIONAL IMAGING IS ABORTED.\nTHIS CASE SHOULD ONLY BE CALLED THEN"
      n62 = global read "General Globals.vi" "Timelapse frames saved"() -> (w147:u32)
      n63 = global read "General Globals.vi" "Protocol start timestamp"() -> (w140:timestamp)
      n64 = Get Date/Time In Seconds() -> (seconds since 1Jan1904=w141:timestamp)
      n65 = call "Experiment header-Calculate STATS.vi"("Logging queue element"=w146, "Timelapse frames saved"=w147) -> ("Number of acquired frames"=w142:dbl, "Acquisition time (ms)"=w143:dbl, "Total number of points acquired (Ch0)"=w144:dbl)  [unwired: 7 in]
      n66 = Subtract(x=w141, y=w140) -> (x-y=w139:dbl)
      n67 = Bundle By Name(cluster=T20 {"Z-stack duration (sec)"=0.0, "Number of acquired data-points"=0.0, "Acquisition time (ms)"=0.0, "Number of acquired frames"=0.0, "Intertrial times"=[]} ("STATISTICS"), "Z-stack duration (sec)"=w139, "Number of acquired data-points"=w144, "Acquisition time (ms)"=w143, "Number of acquired frames"=w142) -> (w138:T20)
      n68 = Bundle By Name(cluster=T6 {"LOGIN"={"User"="Olympus  20X", "Profile"="", "Software Version"="", "Experiment Date Time"=timestamp(0 s since 1904-01-01)}, "GLOBAL PARAMETERS"={"MicroscopeID"="", "Microscope Type"="", "Objective"="", "Field of View (um)"=0.0, "Fill time (us)"=0.0, "Experiment Type"=enum."In vivo", "Stimuli Trigger"=FALSE, "Speed Logging"=FALSE}, "IMAGING MODES"={"Time Series"=FALSE, "Motor Zstack"=FALSE, "AOL Zstack"=FALSE, "Functional Imaging"=FALSE, "Volume Imaging"=FALSE}, "TIME SERIES"={"Basic Image meta data"={"Wavelength (nm)"=0.0, "# averaged frames"=0.0, "laser power (%)"=0.0, "Pockels"=0.0, "pixel dwell time (us)"=0.0, "pmt 1"=0.0, "pmt 2"=0.0, "back apperture"=0.0, "zoom"=0.0, "field of view"=0.0, "Frame Size"=0, "AOL x centre"=0.0, "AOL y centre"=0.0, "Stage x position"=0.0, "Stage y position"=0.0, "Stage z position"=0.0}, "AOL z"=0.0}, "MOTOR Z-STACK "={"Hdr Basic Image meta data"={"Wavelength (nm)"=0.0, "# averaged frames"=0.0, "laser power (%)"=0.0, "Pockels"=0.0, "pixel dwell time (us)"=0.0, "pmt 1"=0.0, "pmt 2"=0.0, "back apperture"=0.0, "zoom"=0.0, "field of view"=0.0, "Frame Size"=0, "AOL x centre"=0.0, "AOL y centre"=0.0, "Stage x position"=0.0, "Stage y position"=0.0, "Stage z position"=0.0}, "Z Start"=0.0, "Z Stop"=0.0, "No of Planes"=0}, "AOL Z-STACK"={"Hdr Basic Image meta data"={"Wavelength (nm)"=0.0, "# averaged frames"=0.0, "laser power (%)"=0.0, "Pockels"=0.0, "pixel dwell time (us)"=0.0, "pmt 1"=0.0, "pmt 2"=0.0, "back apperture"=0.0, "zoom"=0.0, "field of view"=0.0, "Frame Size"=0, "AOL x centre"=0.0, "AOL y centre"=0.0, "Stage x position"=0.0, "Stage y position"=0.0, "Stage z position"=0.0}, "Z Start"=0.0, "Z Stop"=0.0, "No of Planes"=0}, "FUNCTIONAL IMAGING"={"Functional Mode"=enum."Point", "Pockels Modulation"=FALSE, "Number of pois"=0.0, "Number of miniscans"=0.0, "Number of cycles"=0.0, "Number of trials"=0.0, "Miniscan dwell time per pixel (us)"=0.0, "Number of pixels in miniscan"=0.0, "poi dwell time"=0.0, "Rectangle ROI length"=0.0, "Rectangle ROI height"=0.0, "AOL Mode"=enum."Raster", "Plane Mode"=0, "video length (sec)"=0.0, "Frame rate (fps)"=0.0, "Stimuli Timing (usec)"=0.0, "Acquisition Length"=0.0, "Basic Image meta data"={"Wavelength (nm)"=0.0, "# averaged frames"=0.0, "laser power (%)"=0.0, "Pockels"=0.0, "pixel dwell time (us)"=0.0, "pmt 1"=0.0, "pmt 2"=0.0, "back apperture"=0.0, "zoom"=0.0, "field of view"=0.0, "Frame Size"=0, "AOL x centre"=0.0, "AOL y centre"=0.0, "Stage x position"=0.0, "Stage y position"=0.0, "Stage z position"=0.0}, "Z Start (um)"=0.0, "Z Stop (um)"=0.0}, "VOLUME IMAGING"={"Functional Mode"=enum."Point", "Pockels Modulation"=FALSE, "Number of pois"=0.0, "Number of miniscans"=0.0, "Number of cycles"=0.0, "Number of trials"=0.0, "Miniscan dwell time per pixel (us)"=0.0, "Number of pixels in miniscan"=0.0, "poi dwell time"=0.0, "Rectangle ROI length"=0.0, "Rectangle ROI height"=0.0, "AOL Mode"=enum."Raster", "Plane Mode"=0, "video length (sec)"=0.0, "Frame rate (fps)"=0.0, "Stimuli Timing (usec)"=0.0, "Acquisition Length"=0.0, "Basic Image meta data"={"Wavelength (nm)"=0.0, "# averaged frames"=0.0, "laser power (%)"=0.0, "Pockels"=0.0, "pixel dwell time (us)"=0.0, "pmt 1"=0.0, "pmt 2"=0.0, "back apperture"=0.0, "zoom"=0.0, "field of view"=0.0, "Frame Size"=0, "AOL x centre"=0.0, "AOL y centre"=0.0, "Stage x position"=0.0, "Stage y position"=0.0, "Stage z position"=0.0}, "Z Start (um)"=0.0, "Z Stop (um)"=0.0}, "CALIBRATION"={"Pockels Calibration File"=path "", "Calibration_ini file"=path "", "Setup_ini file"=path ""}, "STATISTICS"={"Z-stack duration (sec)"=0.0, "Number of acquired data-points"=0.0, "Acquisition time (ms)"=0.0, "Number of acquired frames"=0.0, "Intertrial times"=[]}, "BIOLOGY INFORMATION"={"Animal Code or Name"="", "Animal DoB"="", "Animal Age"="", "Animal Sex"="", "Animal Weight"="", "Date of Injection"="", "Date of Implant"="", "Site of Injection"="", "Animal Ear Notch"="", "AAV constructs"="", "Genetic background"="", "Optical reporter"="", "Region of brain imaged"="", "Other \ncomments"=""}} ("All header parameters in"), "STATISTICS"=w138) -> (w148:T6)
    }
    frame "BIOLOGY INFORMATION" {
      n69 = global read "gl_UI Ctrl Refs.vi" "UI ctrl refs"() -> (w154:T24)
      n70 = Unbundle By Name(w154) -> ("Biology Information"=w153:refnum<vi>)
      n71 = property class="Clust (strict)"(reference=w153) -> ("Value"=w151:T21)  [unwired: 1 in, 2 out]
      n72 = Bundle By Name(cluster=T6 {"LOGIN"={"User"="Olympus  20X", "Profile"="", "Software Version"="", "Experiment Date Time"=timestamp(0 s since 1904-01-01)}, "GLOBAL PARAMETERS"={"MicroscopeID"="", "Microscope Type"="", "Objective"="", "Field of View (um)"=0.0, "Fill time (us)"=0.0, "Experiment Type"=enum."In vivo", "Stimuli Trigger"=FALSE, "Speed Logging"=FALSE}, "IMAGING MODES"={"Time Series"=FALSE, "Motor Zstack"=FALSE, "AOL Zstack"=FALSE, "Functional Imaging"=FALSE, "Volume Imaging"=FALSE}, "TIME SERIES"={"Basic Image meta data"={"Wavelength (nm)"=0.0, "# averaged frames"=0.0, "laser power (%)"=0.0, "Pockels"=0.0, "pixel dwell time (us)"=0.0, "pmt 1"=0.0, "pmt 2"=0.0, "back apperture"=0.0, "zoom"=0.0, "field of view"=0.0, "Frame Size"=0, "AOL x centre"=0.0, "AOL y centre"=0.0, "Stage x position"=0.0, "Stage y position"=0.0, "Stage z position"=0.0}, "AOL z"=0.0}, "MOTOR Z-STACK "={"Hdr Basic Image meta data"={"Wavelength (nm)"=0.0, "# averaged frames"=0.0, "laser power (%)"=0.0, "Pockels"=0.0, "pixel dwell time (us)"=0.0, "pmt 1"=0.0, "pmt 2"=0.0, "back apperture"=0.0, "zoom"=0.0, "field of view"=0.0, "Frame Size"=0, "AOL x centre"=0.0, "AOL y centre"=0.0, "Stage x position"=0.0, "Stage y position"=0.0, "Stage z position"=0.0}, "Z Start"=0.0, "Z Stop"=0.0, "No of Planes"=0}, "AOL Z-STACK"={"Hdr Basic Image meta data"={"Wavelength (nm)"=0.0, "# averaged frames"=0.0, "laser power (%)"=0.0, "Pockels"=0.0, "pixel dwell time (us)"=0.0, "pmt 1"=0.0, "pmt 2"=0.0, "back apperture"=0.0, "zoom"=0.0, "field of view"=0.0, "Frame Size"=0, "AOL x centre"=0.0, "AOL y centre"=0.0, "Stage x position"=0.0, "Stage y position"=0.0, "Stage z position"=0.0}, "Z Start"=0.0, "Z Stop"=0.0, "No of Planes"=0}, "FUNCTIONAL IMAGING"={"Functional Mode"=enum."Point", "Pockels Modulation"=FALSE, "Number of pois"=0.0, "Number of miniscans"=0.0, "Number of cycles"=0.0, "Number of trials"=0.0, "Miniscan dwell time per pixel (us)"=0.0, "Number of pixels in miniscan"=0.0, "poi dwell time"=0.0, "Rectangle ROI length"=0.0, "Rectangle ROI height"=0.0, "AOL Mode"=enum."Raster", "Plane Mode"=0, "video length (sec)"=0.0, "Frame rate (fps)"=0.0, "Stimuli Timing (usec)"=0.0, "Acquisition Length"=0.0, "Basic Image meta data"={"Wavelength (nm)"=0.0, "# averaged frames"=0.0, "laser power (%)"=0.0, "Pockels"=0.0, "pixel dwell time (us)"=0.0, "pmt 1"=0.0, "pmt 2"=0.0, "back apperture"=0.0, "zoom"=0.0, "field of view"=0.0, "Frame Size"=0, "AOL x centre"=0.0, "AOL y centre"=0.0, "Stage x position"=0.0, "Stage y position"=0.0, "Stage z position"=0.0}, "Z Start (um)"=0.0, "Z Stop (um)"=0.0}, "VOLUME IMAGING"={"Functional Mode"=enum."Point", "Pockels Modulation"=FALSE, "Number of pois"=0.0, "Number of miniscans"=0.0, "Number of cycles"=0.0, "Number of trials"=0.0, "Miniscan dwell time per pixel (us)"=0.0, "Number of pixels in miniscan"=0.0, "poi dwell time"=0.0, "Rectangle ROI length"=0.0, "Rectangle ROI height"=0.0, "AOL Mode"=enum."Raster", "Plane Mode"=0, "video length (sec)"=0.0, "Frame rate (fps)"=0.0, "Stimuli Timing (usec)"=0.0, "Acquisition Length"=0.0, "Basic Image meta data"={"Wavelength (nm)"=0.0, "# averaged frames"=0.0, "laser power (%)"=0.0, "Pockels"=0.0, "pixel dwell time (us)"=0.0, "pmt 1"=0.0, "pmt 2"=0.0, "back apperture"=0.0, "zoom"=0.0, "field of view"=0.0, "Frame Size"=0, "AOL x centre"=0.0, "AOL y centre"=0.0, "Stage x position"=0.0, "Stage y position"=0.0, "Stage z position"=0.0}, "Z Start (um)"=0.0, "Z Stop (um)"=0.0}, "CALIBRATION"={"Pockels Calibration File"=path "", "Calibration_ini file"=path "", "Setup_ini file"=path ""}, "STATISTICS"={"Z-stack duration (sec)"=0.0, "Number of acquired data-points"=0.0, "Acquisition time (ms)"=0.0, "Number of acquired frames"=0.0, "Intertrial times"=[]}, "BIOLOGY INFORMATION"={"Animal Code or Name"="", "Animal DoB"="", "Animal Age"="", "Animal Sex"="", "Animal Weight"="", "Date of Injection"="", "Date of Implant"="", "Site of Injection"="", "Animal Ear Notch"="", "AAV constructs"="", "Genetic background"="", "Optical reporter"="", "Region of brain imaged"="", "Other \ncomments"=""}} ("All header parameters in"), "BIOLOGY INFORMATION"=w151) -> (w150:T6)
    }
  }
  "All header parameters in" <- w6
  n73 = case shown="True" "Update header\ninterface cluster ?" {
    tunnel: w6 -> [_ w159]
    tunnel: "error in (no error)" -> [w155 w158]
    tunnel: [w155 w157] -> w4
    tunnel: "Header file sections" -> [_ w156]
    frame False {
    }
    frame True {
      n74 = call "Experiment header-Interface module.vi"("Header file sections"=w156, "error in (no error)"=w158, "All header parameters in"=w159, "Function"=Header_file_interface_module_functions_enum."Update values in memory") -> ("error out"=w157:errorcluster)  [unwired: 6 in, 1 out]
    }
  }
  "error out" <- w4
